vi "Automatic_IV_CV_with_XML_Global_Stop_V1.0.vi"() -> ()   [LabVIEW 2009]
uses:
  subVIs/CMSFPIX_LV80.llb/Keith 237 Operate/Standby.vi
  <vilib>/xml/Close Reference(Node).vi
  <vilib>/Utility/file.llb/Write To Spreadsheet File (string).vi
  <vilib>/Utility/file.llb/Write To Spreadsheet File (DBL).vi
  <vilib>/xml/NI_XML.lvlib
panel:
  out "voltage \ncompliance level":dbl=1e-05
  out "Wafer Number":string
  out "Contact Check Result":string="Skipped"
  out "Site Number":i32
  out "File Name":string
  in  "Tab Control 2":enum32{"IV Check", "CV Check"}(tab)
  out "Boolean":bool caption="Voltage Breakdown"
  out "Boolean 2":bool caption="Leakage Current Check Total"
  out "Boolean 3":bool caption="Leakage Current Check Active"
  out "Boolean 4":bool caption="Leakage Current Check Guardring"
  out "Boolean 5":bool caption="150V Bias Check"
  out "Contact Check":bool
  out "Status":string
  out "Bias Polarity":dbl=1.0 format="%.2f"
  out "1/C^2":cluster{"Y":dbl[], "Y":dbl[]}[](graph)
  out "semaphore":T1
  out "voltage \ncompliance cutoff":dbl=1e-05
  in  "Tab Control":enum32{"Site Selection"}(tab)
  in  "Site 1":bool=TRUE
  in  "Site 2":bool=TRUE
  in  "Site 3":bool=TRUE
  in  "Site 4":bool=TRUE
  in  "Site 5":bool=TRUE
  in  "Site 6":bool=TRUE
  in  "Site 7":bool=TRUE
  in  "Site 8":bool=TRUE
  in  "Site 9":bool=TRUE
  in  "Site 10":bool=TRUE
  in  "Site 11":bool=TRUE
  in  "Site 12":bool=TRUE
  in  "Site 13":bool=TRUE
  in  "Site 14":bool=TRUE
  in  "Site 15":bool=TRUE
  in  "Site 16":bool=TRUE
  in  "Site 17":bool=TRUE
  in  "Site 18":bool=TRUE
  in  "Site 19":bool=TRUE
  in  "Site 20":bool=TRUE
  in  "Site 21":bool=TRUE
  in  "Site 22":bool=TRUE
  in  "Running Conditional":bool
  out "error out 7":T2
  in  "IV or CV":i32
  in  "Emergency Stop":bool
  out "error out 6":T2
  in  "Stop Loop":bool=TRUE
  in  "Total Site # CV":i32=12
  out "Secondary Parameter":u16(ring) items=["None", "Cs", "Cp", "Ls", "Lp", "Rs", "Rp", "DF", "Q", "Z", "Y", "Phase", "ESR", "Gp", "Xs", "Bp"]
  out "Auto Compliance":dbl=9.9e-05
  out "Compliance":dbl=1e-09
  out "Compliance":bool
  out "Compliance Level":dbl format="%#_6e"
  out "Secondary Parameter Graph":cluster{"Y":dbl[], "Y":dbl[]}[](graph) caption="DF"
  in  "Absolute?":bool
  out "Voltage Range":string
  out "Primary Parameter":u16(ring)=2 items=["AUTO", "Cs", "Cp", "Ls", "Lp", "Rs", "Rp", "DF", "Q", "Z", "Y", "Phase", "ESR", "Gp", "Xs", "Bp"]
  out "Time Delay mS":dbl=20.0
  out "Number of Averages":dbl=1.0
  out "Voltage Level":dbl=1.0
  out "Frequency":dbl=1000.0
  in  "Bias Loop":bool
  out "K237_Bias":dbl
  in  "Archive":T3(tab)=enum."Primary"
  out "Diode Total Current Archive":cluster{"Y":dbl[], "Y":dbl[]}[](graph) caption="Total Current"
  out "Diode GRD Archive":cluster{"Y":dbl[], "Y":dbl[]}[](graph)
  out "Diode ACTIVE Archive":cluster{"Y":dbl[], "Y":dbl[]}[](graph)
  out "Single Chip Total Current Archive":cluster{"Y":dbl[], "Y":dbl[]}[](graph) caption="Total Current"
  out "Single Chip GRD Archive":cluster{"Y":dbl[], "Y":dbl[]}[](graph)
  out "Single Chip ACTIVE Archive":cluster{"Y":dbl[], "Y":dbl[]}[](graph)
  out "2x8 Total Current Archive":cluster{"Y":dbl[], "Y":dbl[]}[](graph) caption="Total Current"
  out "2x8 GRD Archive":cluster{"Y":dbl[], "Y":dbl[]}[](graph)
  out "2x8 ACTIVE Archive":cluster{"Y":dbl[], "Y":dbl[]}[](graph)
  out "Slim-Edge ACTIVE Archive":cluster{"Y":dbl[], "Y":dbl[]}[](graph)
  out "Slim-Edge GRD Archive":cluster{"Y":dbl[], "Y":dbl[]}[](graph)
  out "Slim-Edge Total Current Archive":cluster{"Y":dbl[], "Y":dbl[]}[](graph) caption="Total Current"
  out "Single Chip Capacitance":cluster{"Y":dbl[], "Y":dbl[]}[](graph)
  out "2x8 Chip Capacitance":cluster{"Y":dbl[], "Y":dbl[]}[](graph)
  out "Diodes Capacitance":cluster{"Y":dbl[], "Y":dbl[]}[](graph)
  in  "Halt CV":bool
  in  "Halt IV":bool
  out "Running?":bool
  in  "Total Site # IV":i32=22
  out "Site # CV":dbl
  out "Site # IV":dbl
  out "error out":errorcluster
  in  "CV-V-Limit":i32=10
  out "Capacitance":cluster{"Y":dbl[], "Y":dbl[]}[](graph) caption="Cp"
  in  "CV-V-Steps":i32=1
  out "QuadTech Status":string
  out "Total Current":cluster{"Y":dbl[], "Y":dbl[]}[](graph)
  out "6485 GRD (GPIB 10)":cluster{"Y":dbl[], "Y":dbl[]}[](graph)
  out "6485 ACTIVE (GPIB 14)":cluster{"Y":dbl[], "Y":dbl[]}[](graph)
  out "error out 5":errorcluster
  out "error out 4":errorcluster
  in  "IV-V-Steps":i32=1
  in  "IV-V-Limit":i32=10
  in  "error in (no error)":errorcluster
  # "Note: The Total Site # indexes\nstarting at 0 and goes to n-1,\nso if there are a total of 3 sites\nthen Total Site # should be set\nto 3"
  # "Note 2: This code is setup for a specific\nwafer map. If a map with a different\nnumber of subsites and/or different layout\nis used the naming will be incorrect"
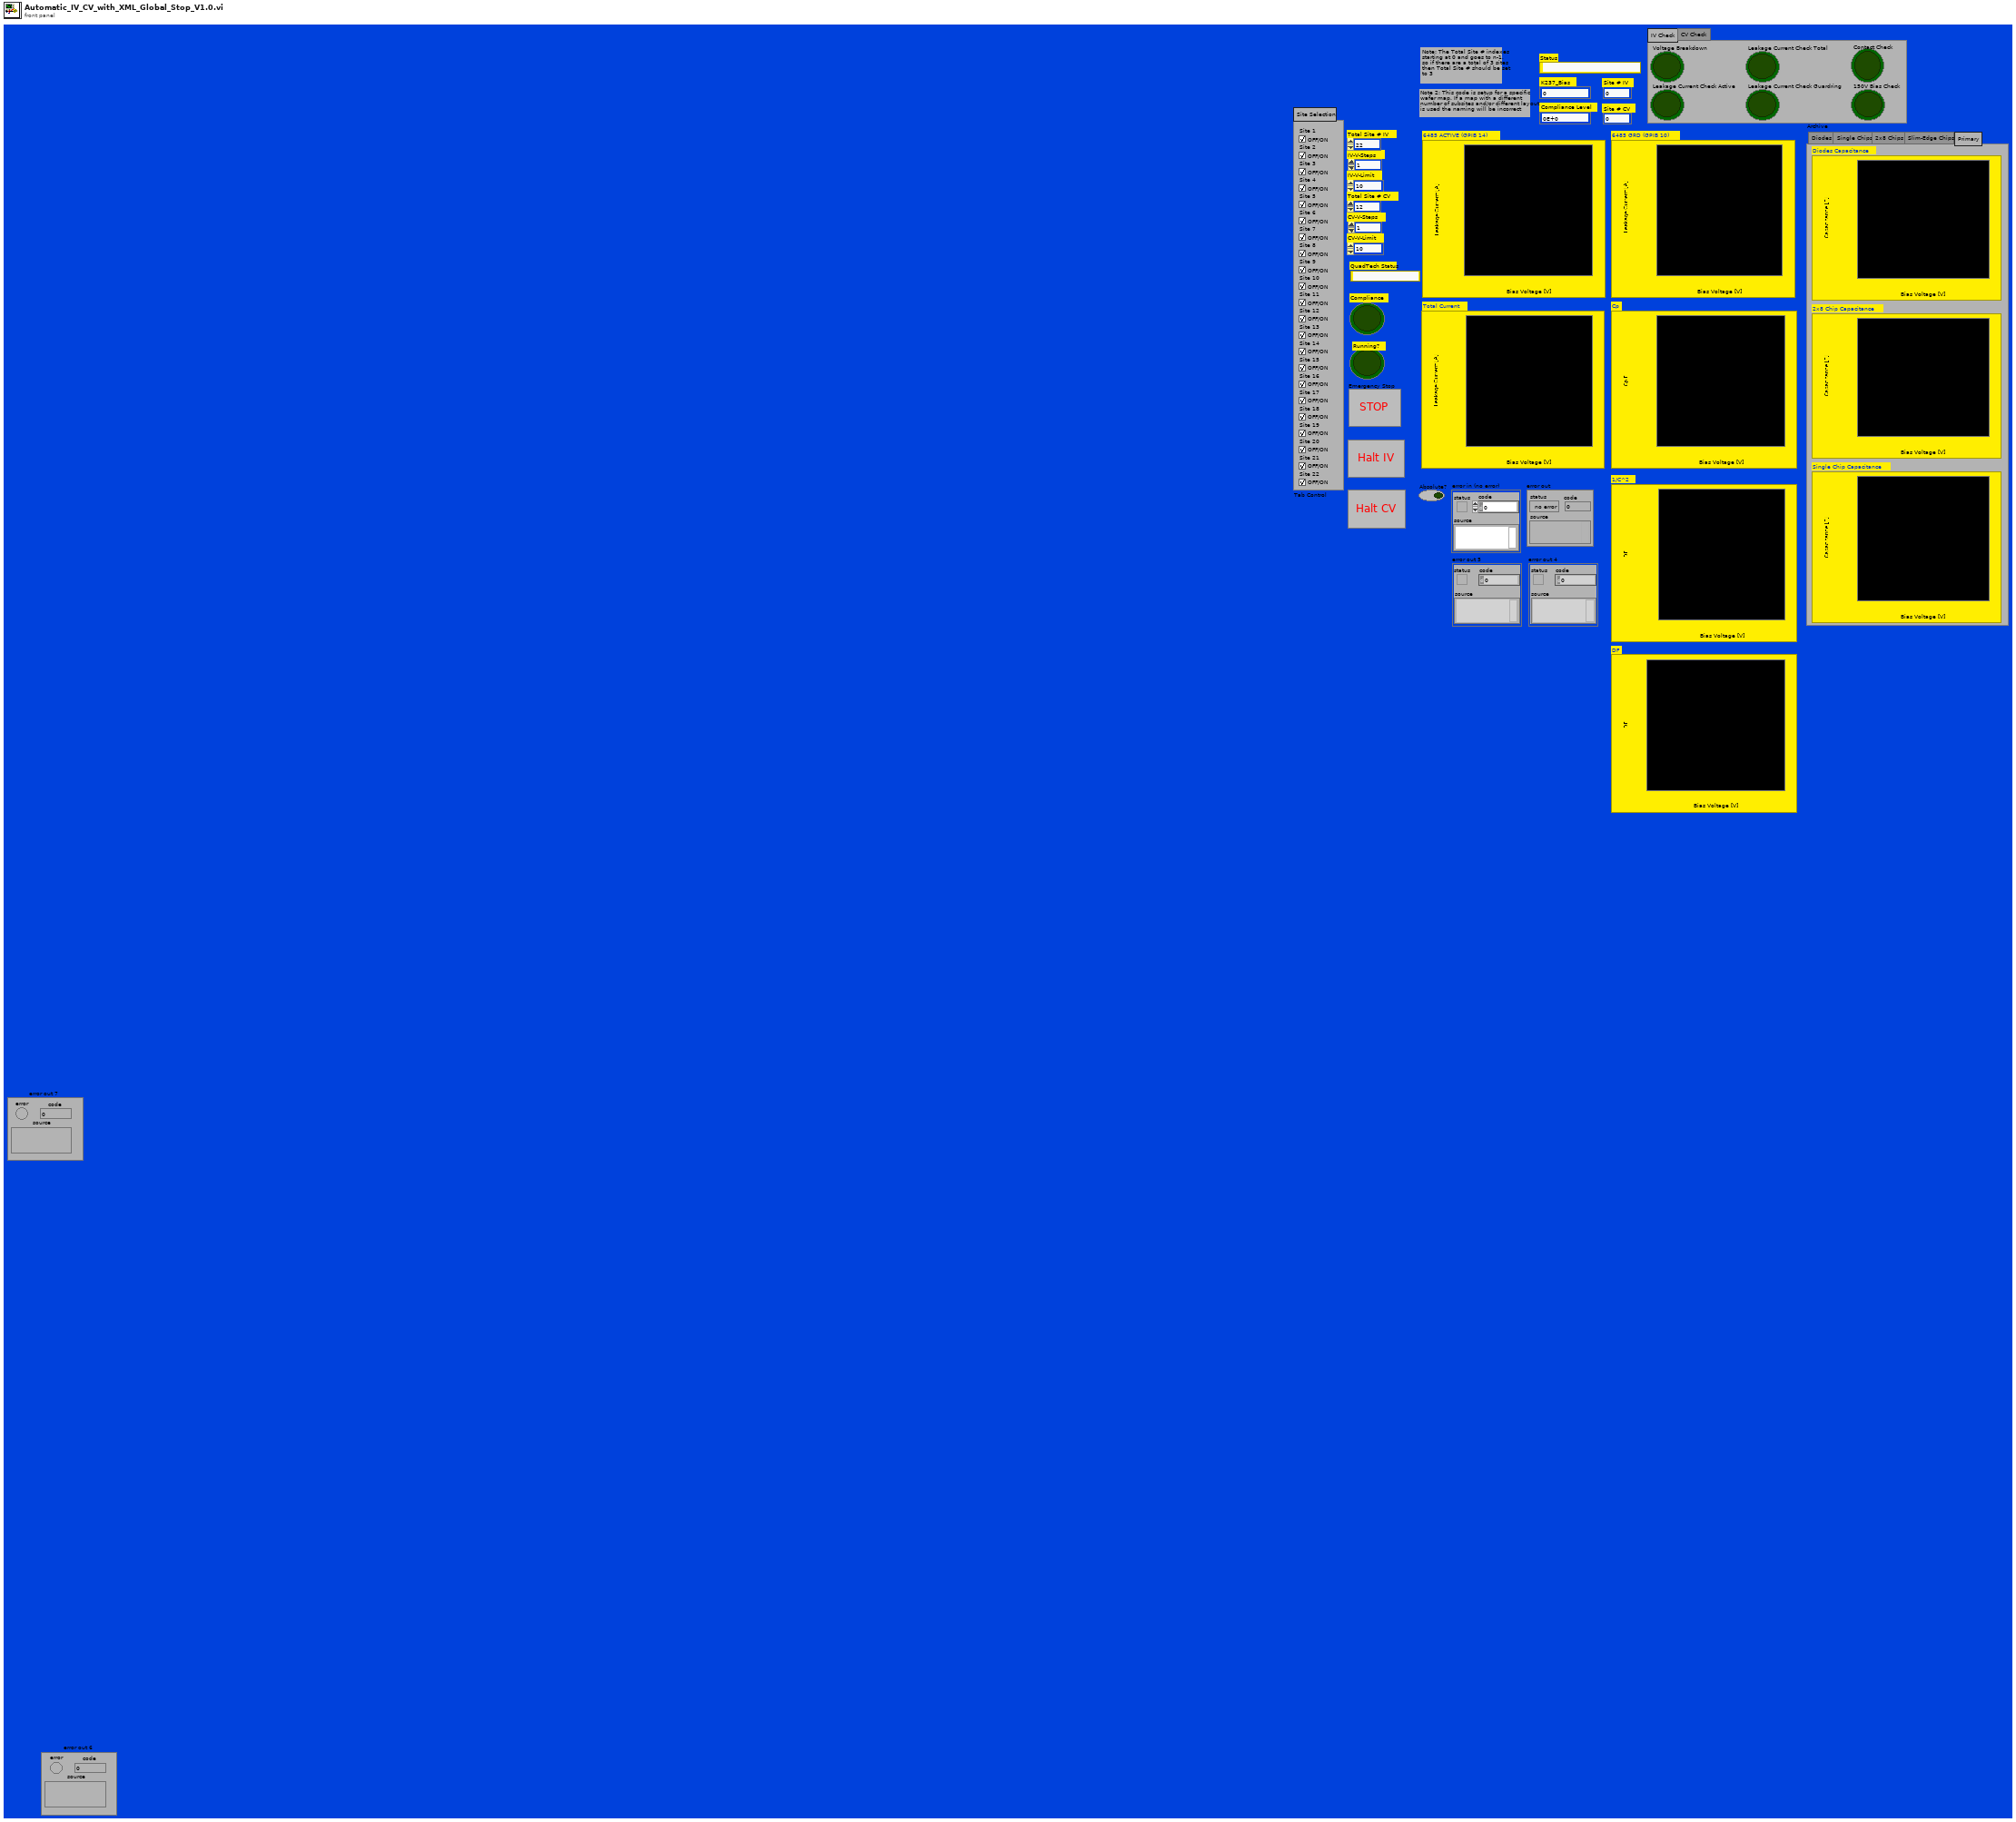
[diagram p1: front panel]
types:
  T1 = typedef "Semaphore RefNum" = refnum<k1>
  T2 = cluster{"error":bool, "code":i32, "source":string}
  T3 = enum32{"Diodes", "Single Chips", "2x8 Chips", "Slim-Edge Chips", "Primary"}
  T4 = cluster{"Name of Test":string, string, "Comment Description":string, "User":string}
  T5 = enum16{"open", "replace", "create", "open or create", "replace or create", "replace or create with confirmation"}
  T6 = cluster{cluster{"Y":dbl[], "Y":dbl[]}[], cluster{"Y":dbl[], "Y":dbl[]}[], cluster{"Y":dbl[], "Y":dbl[]}[], cluster{"Y":dbl[], "Y":dbl[]}[], cluster{"Y":dbl[], "Y":dbl[]}[], cluster{"Y":dbl[], "Y":dbl[]}[], cluster{"Y":dbl[], "Y":dbl[]}[], cluster{"Y":dbl[], "Y":dbl[]}[], cluster{"Y":dbl[], "Y":dbl[]}[], cluster{"Y":dbl[], "Y":dbl[]}[], cluster{"Y":dbl[], "Y":dbl[]}[], cluster{"Y":dbl[], "Y":dbl[]}[]}
  T7 = enum16{"Left Button", "Center Button", "Right Button", "Window Close"}
  T8 = cluster{"error":bool, "code":i8, "source":string}
  T9 = cluster{cluster{"Y":dbl[], "Y":dbl[]}[], cluster{"Y":dbl[], "Y":dbl[]}[], cluster{"Y":dbl[], "Y":dbl[]}[]}
  T10 = cluster{"Primary ":string, "Primary Value":string, "Primary Unit":string, "Secondary":string, "Secondary Value":string, "Secondary Unit":string}
  T11 = cluster{"XY Graph":cluster{"Y":dbl[], "Y":dbl[]}[], "XY Graph":cluster{"Y":dbl[], "Y":dbl[]}[], "XY Graph":cluster{"Y":dbl[], "Y":dbl[]}[]}
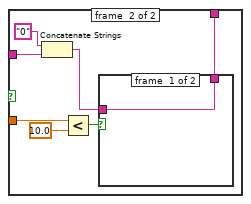
[diagram p4: hidden frame]
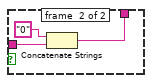
[diagram p5: hidden frame]
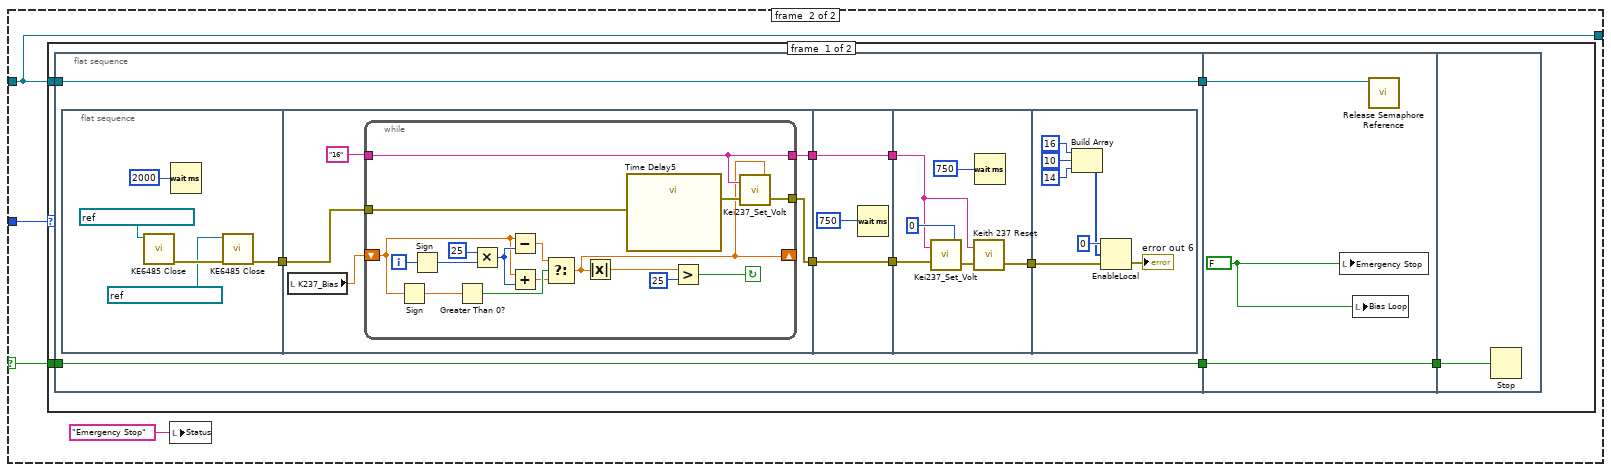
[diagram p7: hidden frame]
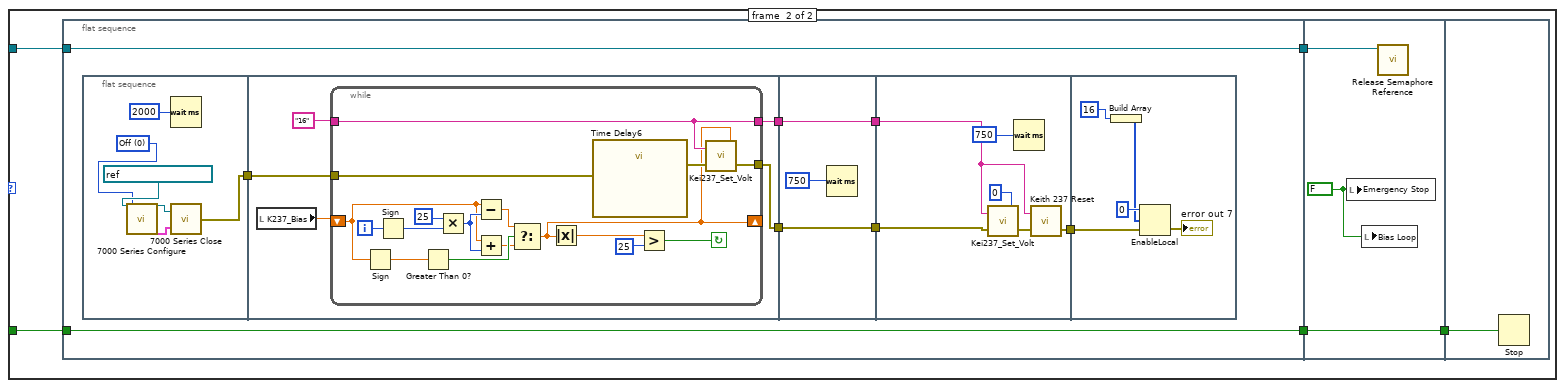
[diagram p8: hidden frame]
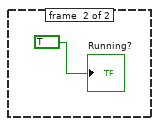
[diagram p9: hidden frame]
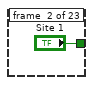
[diagram p10: hidden frame]
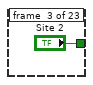
[diagram p11: hidden frame]
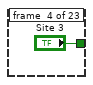
[diagram p12: hidden frame]
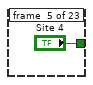
[diagram p13: hidden frame]
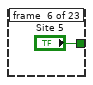
[diagram p14: hidden frame]
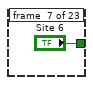
[diagram p15: hidden frame]
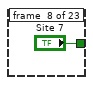
[diagram p16: hidden frame]
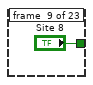
[diagram p17: hidden frame]
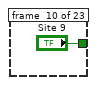
[diagram p18: hidden frame]
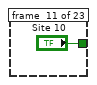
[diagram p19: hidden frame]
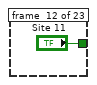
[diagram p20: hidden frame]
diagram:
  (unwired) path "" ("base path")
  # "Wafer Folder"
  # "Test Name Subfolder"
  # "XML Subfolder"
  # "Single Chip"
  # "2x8"
  # "Diode"
  # "Total"
  # "GRD"
  # "Active"
  # "Capacitance"
  # "Slim-Edge"
  # "2x8"
  # "Single Chip"
  # "Diodes"
  # "Change wiring to CV"
  # "DO CV MEASUREMENTS"
  # "Do CV measurements"
  # "Configure CV instuments"
  # "Do IV measurements"
  # "Configure IV instuments"
  # "DO IV MEASUREMENTS"
  n1 = invoke on="Diode ACTIVE Archive" class="XYGraph (strict)" method="Reinit To Default"() -> ()  [unwired: 3 in, 3 out]
  n2 = invoke on="Diode GRD Archive" class="XYGraph (strict)" method="Reinit To Default"() -> ()  [unwired: 3 in, 3 out]
  n3 = invoke on="Diode Total Current Archive" class="XYGraph (strict)" method="Reinit To Default"() -> ()  [unwired: 3 in, 3 out]
  n4 = invoke on="Diodes Capacitance" class="XYGraph (strict)" method="Reinit To Default"() -> ()  [unwired: 3 in, 3 out]
  n5 = invoke on="2x8 Chip Capacitance" class="XYGraph (strict)" method="Reinit To Default"() -> ()  [unwired: 3 in, 3 out]
  n6 = invoke on="Single Chip Capacitance" class="XYGraph (strict)" method="Reinit To Default"() -> ()  [unwired: 3 in, 3 out]
  n7 = invoke on="Single Chip ACTIVE Archive" class="XYGraph (strict)" method="Reinit To Default"() -> ()  [unwired: 3 in, 3 out]
  n8 = invoke on="Single Chip GRD Archive" class="XYGraph (strict)" method="Reinit To Default"() -> ()  [unwired: 3 in, 3 out]
  n9 = invoke on="Single Chip Total Current Archive" class="XYGraph (strict)" method="Reinit To Default"() -> ()  [unwired: 3 in, 3 out]
  n10 = invoke on="2x8 ACTIVE Archive" class="XYGraph (strict)" method="Reinit To Default"() -> ()  [unwired: 3 in, 3 out]
  n11 = invoke on="2x8 GRD Archive" class="XYGraph (strict)" method="Reinit To Default"() -> ()  [unwired: 3 in, 3 out]
  n12 = invoke on="2x8 Total Current Archive" class="XYGraph (strict)" method="Reinit To Default"() -> ()  [unwired: 3 in, 3 out]
  n13 = local write "K237_Bias"(0.0 ("K237_Bias")) -> ()
  n14 = invoke on="Slim-Edge ACTIVE Archive" class="XYGraph (strict)" method="Reinit To Default"() -> ()  [unwired: 3 in, 3 out]
  n15 = invoke on="Slim-Edge GRD Archive" class="XYGraph (strict)" method="Reinit To Default"() -> ()  [unwired: 3 in, 3 out]
  n16 = invoke on="Slim-Edge Total Current Archive" class="XYGraph (strict)" method="Reinit To Default"() -> ()  [unwired: 3 in, 3 out]
  n17 = call "Wafer ID"("error in (no error)"="error in (no error)") -> ("User"=w20:string, "Comment Description"=w21:string, "Name of Test"=w3:string, "Wafer ID #"=w14:dbl, "OK"=w62:bool, "error out"=w65:errorcluster)  [unwired: 13 in]
  n18 = Number To Decimal String(number=w14) -> (decimal integer string=w15:string)  [unwired: 1 in]
  n19 = Less?(x=w14, y=100.0) -> (x < y?=w17:bool)
  n20 = case shown="True" w17 {
    tunnel: w15 -> [w67 w74]
    tunnel: w14 -> [_ w71]
    tunnel: [w67 w68] -> w13
    frame #0 {
    }
    frame #1 {
      n21 = Concatenate Strings("0" ("string"), w74) -> (w69:string)
      n22 = Less?(x=w71, y=10.0) -> (x < y?=w72:bool)
      n23 = case shown="True" w72 {
        tunnel: w69 -> [w75 w78]
        tunnel: [w75 w76] -> w68
        frame #0 {
        }
        frame #1 {
          n24 = Concatenate Strings("0" ("string"), w78) -> (w76:string)
        }
      }
    }
  }
  "Wafer Number" <- w13
  n25 = Not(x=w62) -> (.not. x?=w61:bool)
  n26 = call <vilib>:"Obtain Semaphore Reference.vi"("size (1)"=1) -> ("semaphore"=w34:T1)  [unwired: 4 in, 2 out]
  "semaphore" <- w34
  n27 = Stop(stop? (T)=w61) -> ()
  n28 = Concatenate Strings("Wafer_" ("string"), w13) -> (w25:string)
  n29 = Build Path(base path=path "C:/Documents and Settings/PROBER/Desktop/Andrew_Test/VI Test Output", name or relative path=w25) -> (appended path=w24:path)
  n30 = Bundle("Name of Test"=w3, w13, "Comment Description"=w21, "User"=w20) -> (w12:T4)  [unwired: 1 in]
  n31 = flat-sequence {
    tunnel: w65 -> [w99]
    tunnel: [w97] -> w64
    tunnel: [w85] -> w58
    tunnel: [w87] -> w57
    tunnel: [w86] -> w56
    tunnel: [w90] -> w35
    tunnel: w34 -> [w90]
    tunnel: [w80] -> w18
    tunnel: w64 -> [w138]
    tunnel: w1 -> [w133]
    tunnel: w58 -> [w131]
    tunnel: w57 -> [w130]
    tunnel: w56 -> [w129]
    tunnel: [w128] -> w45
    tunnel: w35 -> [w121]
    tunnel: [w120] -> w28
    tunnel: w12 -> [w119]
    tunnel: w18 -> [w118]
    tunnel: w1 -> [w113]
    tunnel: w7 -> [w111]
    tunnel: w45 -> [w1215]
    tunnel: [w1215] -> w44
    tunnel: [w1213] -> w29
    tunnel: w28 -> [w1213]
    tunnel: [w1219] -> w46
    tunnel: w44 -> [w1220]
    tunnel: [w1217] -> w30
    tunnel: w29 -> [w1217]
    tunnel: w46 -> [w1229]
    tunnel: [w1229] -> w63
    tunnel: [w1225] -> w31
    tunnel: w30 -> [_]
    tunnel: w63 -> [w1238]
    tunnel: [w1237] -> w55
    tunnel: [w1236] -> w53
    tunnel: [w1235] -> w51
    tunnel: [w1233] -> w49
    tunnel: [w1232] -> w32
    tunnel: w31 -> [w1232]
    tunnel: w55 -> [w1272]
    tunnel: [w1272] -> w54
    tunnel: w53 -> [w1271]
    tunnel: [w1271] -> w52
    tunnel: w51 -> [w1270]
    tunnel: [w1270] -> w50
    tunnel: w49 -> [w1269]
    tunnel: ["Total Site # CV"] -> w37
    tunnel: [w1267] -> w33
    tunnel: w32 -> [w1267]
    tunnel: w54 -> [w1320]
    tunnel: w52 -> [w1319]
    tunnel: w50 -> [w1318]
    tunnel: w1 -> [w1310]
    tunnel: [FALSE ("Compliance")] -> w43
    tunnel: [TRUE ("Bias Loop")] -> w41
    tunnel: [w1308] -> w39
    tunnel: w37 -> [w1307]
    tunnel: w33 -> [w1306]
    tunnel: w12 -> [w1304]
    tunnel: w7 -> [w1303]
    tunnel: w43 -> [w1874]
    tunnel: [w1874] -> w42
    tunnel: w41 -> [w1877]
    tunnel: [w1877] -> w40
    tunnel: w39 -> [w1876]
    tunnel: [w1876] -> w38
    tunnel: [w1885] -> w47
    tunnel: [w1886] -> w48
    tunnel: w42 -> [w1886]
    tunnel: w40 -> [w1885]
    tunnel: w38 -> [w1880]
    frame #0 {
      w80 = 0 ("Numeric")
      w91 = FALSE
      w100 = u16 5 items=["auto / auto", "1 nA / 1.1 V", "10 nA / 11 V", "100 nA / 110 V", "0.001 mA / 1100 V", "0.01 mA / 1100 V", "0.1 mA / 1100 V", "1 mA / 1100 V", "10 mA / 1100 V", "100 mA / 1100 V"] ("source range\nI source / V source (auto:0)")
      w103 = u16 0 items=["voltage/current", "current/voltage"] ("source/measure (V/I:0)")
      w104 = u16 5 items=["auto / auto", "1 nA / 1.1 V", "10 nA / 11 V", "100 nA / 110 V", "0.001 mA / 1100 V", "0.01 mA / 1100 V", "0.1 mA / 1100 V", "1 mA / 1100 V", "10 mA / 1100 V", "100 mA / 1100 V"] ("compliance/\nmeasurement range (auto:0)")
      w102 = 1e-05 ("voltage \ncompliance level")
      w107 = u16 0 items=["DC", "sweep"] ("function (DC:0)")
      w97 = "16"  # GPIB
      # "Change Bias Polarity\n+1 Chuck Bias\n-1  Pad bias"
      # "Keithley 237 as sourcemeter\nKeithley 6485 as picoammeters"
      n32 = call "Keith 237 Reset.vi"("GPIB address"=w97, "error in"=w99) -> ("error out"=w98:T2)
      n33 = call "Keith 237 Basic Config.vi"("GPIB address"=w97, "source/measure (V/I:0)"=w103, "function (DC:0)"=w107, "source range\nI source / V source (auto:0)"=w100, "source level"=0.0, "error in"=w98, "1100 V range (disabled:F)"=TRUE, "current \ncompliance level"=w102, "compliance/\nmeasurement range (auto:0)"=w104) -> ("error out"=w109:T2)  [unwired: 7 in, 3 out]
      n34 = local write "IV or CV"(w80) -> ()
      n35 = call "Keith 237 Operate/Standby.vi"("source"=FALSE, "error in"=w109, "GPIB address"=w97) -> ("error out"=w108:T2)
      n36 = Multiply(x=w102, y=0.98 ("voltage \ncompliance level")) -> (x*y=→"voltage \ncompliance cutoff":dbl)
      n37 = call "Keith 237 Send Trigger.vi"("GPIB address"=w97, "error in"=w108) -> ("error out"=w95:T2)
      n38 = call "KE6485 Initialize.vi"("error in (no error)"=w95, "resource name"=refnum<k15> "GPIB0::10::INSTR" ("instrument handle")) -> ("error out"=w89:errorcluster, "instrument handle out"=w92:refnum<k15>)  [unwired: 8 in]
      n39 = property class="KE6485"(reference=w92, error in=w89, "System Settings:Zero Check Enabled"=w91) -> (reference out=w85:refnum<k15>, error out=w84:errorcluster)
      n40 = call "KE6485 Initialize.vi"("error in (no error)"=w84, "resource name"=refnum<k15> "GPIB0::14::INSTR" ("instrument handle")) -> ("error out"=w88:errorcluster, "instrument handle out"=w93:refnum<k15>)  [unwired: 8 in]
      n41 = property class="KE6485"(reference=w93, error in=w88, "System Settings:Zero Check Enabled"=w91) -> (reference out=w87:refnum<k15>, error out=w86:errorcluster)
      "Bias Polarity" <- 1.0
      "Status" <- "Setting IV Scan Parameters" ("Status")
      "voltage \ncompliance level" <- w102
    }
    frame #1 {
      w122 = cluster{"Y":dbl[], "Y":dbl[]}[] []
      # "10"
      # "14"
      n42 = Build Path(base path=w113, name or relative path="Contact_Check.csv") -> (appended path=w117:path)
      n43 = Open/Create/Replace File(file path (use dialog)=w117, operation (0:open)=T5."replace or create", access (0:read/write)=enum16{"read/write", "read-only", "write-only"}."read/write") -> (refnum out=w116:refnum<file>)  [unwired: 1 in, 4 out]
      n44 = Refnum to Path(1:w116) -> (0:w112:path)
      n45 = for {
        N: "Total Site # IV" -> [_]
        tunnel: w138 -> [w232]
        tunnel: "IV-V-Limit" -> [w234]
        tunnel: "IV-V-Steps" -> [w235]
        tunnel: [w231] -> w136
        shift-right: [w230] -> w124
        shift-left: w129 -> [w233]
        shift-right: [w225] -> _
        shift-left: w122 -> [w196]
        shift-right: [w224] -> _
        shift-left: w122 -> [w195]
        shift-right: [w223] -> _
        shift-left: w122 -> [w194]
        shift-right: [w222] -> _
        shift-left: w122 -> [w193]
        shift-right: [w221] -> _
        shift-left: w122 -> [w188]
        shift-right: [w220] -> _
        shift-left: w122 -> [w192]
        shift-right: [w219] -> _
        shift-left: w122 -> [w191]
        shift-right: [w199] -> _
        shift-left: w122 -> [w190]
        shift-right: [w218] -> _
        shift-left: w122 -> [w189]
        tunnel: w133 -> [w201]
        tunnel: "Absolute?" -> [w200]
        tunnel: w131 -> [w198]
        tunnel: w130 -> [w197]
        shift-right: [w183] -> _
        shift-left: w122 -> [w186]
        shift-right: [w182] -> _
        shift-left: w122 -> [w185]
        shift-right: [w181] -> _
        shift-left: w122 -> [w184]
        tunnel: w121 -> [w180]
        tunnel: [w179] -> w120
        tunnel: w119 -> [w164]
        tunnel: w118 -> [w166]
        tunnel: w112 -> [w142]
        tunnel: w111 -> [w140]
        i -> [w165]
        (unwired) TRUE
        # "User Input Array\nElement 0: Comment Description (XML_Header)\nElement 1: Serial Number\nElement 2: Kind of Part\nElement 3: User\nElement 4: Extension Table Name\nElement 5: Comment Description (XML_Data_Set)\nElement 6: Name (XML_Header)\nElement 7: Run Name (XML_Header)"
        # "XML Data Tags for IV scan"
        n46 = Increment(x=w165) -> (x+1=→"Site # IV":i32)
        n47 = Bundle(w196, w195, w194, w193, w192, w191, w190, w189, w188, w186, w185, w184) -> (w187:T6)  [unwired: 1 in]
        n48 = flat-sequence {
          tunnel: [w246] -> w150
          tunnel: w233 -> [w246]
          tunnel: [w245] -> w152
          tunnel: w232 -> [w245]
          tunnel: w165 -> [w237]
          tunnel: [w244] -> w154
          tunnel: w198 -> [w244]
          tunnel: [w243] -> w156
          tunnel: w197 -> [w243]
          tunnel: w180 -> [w242]
          tunnel: [w242] -> w158
          tunnel: [w236] -> w148
          tunnel: [w238] -> w147
          tunnel: [w240] -> w145
          tunnel: [w237] -> w141
          tunnel: w158 -> [w288]
          tunnel: [w287] -> w157
          tunnel: w156 -> [w286]
          tunnel: [w285] -> w155
          tunnel: w154 -> [w284]
          tunnel: [w283] -> w153
          tunnel: w152 -> [w281]
          tunnel: [w280] -> w151
          tunnel: w150 -> [w282]
          tunnel: [w279] -> w149
          tunnel: w148 -> [w271]
          tunnel: w147 -> [w275]
          tunnel: [w275] -> w146
          tunnel: w145 -> [w276]
          tunnel: [w276] -> w144
          tunnel: [w278] -> w143
          tunnel: w141 -> [w272]
          tunnel: w235 -> [w540]
          tunnel: w234 -> [w539]
          tunnel: [w536] -> w207
          tunnel: [w535] -> w206
          tunnel: [w528] -> w205
          tunnel: [w534] -> w204
          tunnel: [w533] -> w203
          tunnel: w217 -> [w532]
          tunnel: w168 -> [w530]
          tunnel: w208 -> [w529]
          tunnel: [w524] -> w202
          tunnel: w200 -> [w527]
          tunnel: [w522] -> w179
          tunnel: w157 -> [w523]
          tunnel: w155 -> [w525]
          tunnel: w153 -> [w526]
          tunnel: w151 -> [w537]
          tunnel: w149 -> [w538]
          tunnel: w146 -> [w517]
          tunnel: w144 -> [w515]
          tunnel: w159 -> [w521]
          tunnel: w139 -> [w520]
          tunnel: w160 -> [w519]
          tunnel: w143 -> [w518]
          tunnel: w139 -> [w513]
          tunnel: w207 -> [w914]
          tunnel: [w913] -> w178
          tunnel: w206 -> [w910]
          tunnel: [w912] -> w176
          tunnel: w205 -> [w917]
          tunnel: [w917] -> w174
          tunnel: w204 -> [w916]
          tunnel: [w916] -> w172
          tunnel: w203 -> [w915]
          tunnel: [w915] -> w170
          tunnel: w202 -> [w911]
          tunnel: w178 -> [w946]
          tunnel: [w946] -> w177
          tunnel: w176 -> [w945]
          tunnel: [w945] -> w175
          tunnel: w174 -> [w944]
          tunnel: [w944] -> w173
          tunnel: w172 -> [w943]
          tunnel: [w943] -> w171
          tunnel: w170 -> [w942]
          tunnel: [w942] -> w169
          tunnel: [w967] -> w230
          tunnel: [w969] -> w231
          tunnel: w177 -> [w969]
          tunnel: w175 -> [w1006]
          tunnel: w165 -> [w1001]
          tunnel: w173 -> [w1000]
          tunnel: w171 -> [w999]
          tunnel: w169 -> [w998]
          tunnel: [w997] -> w225
          tunnel: [w996] -> w224
          tunnel: [w995] -> w223
          tunnel: [w994] -> w222
          tunnel: [w993] -> w221
          tunnel: [w992] -> w220
          tunnel: [w991] -> w219
          tunnel: [w990] -> w199
          tunnel: [w989] -> w218
          tunnel: w187 -> [w987]
          tunnel: [w973] -> w183
          tunnel: [w972] -> w182
          tunnel: [w971] -> w181
          tunnel: w142 -> [w951]
          frame #0 {
            n49 = Increment(x=w237) -> (x+1=w241:i32)
            n50 = case shown="1" w241 {
              tunnel: [TRUE "Site 1" "Site 2" "Site 3" "Site 4" "Site 5" "Site 6" "Site 7" "Site 8" "Site 9" "Site 10" "Site 11" "Site 12" "Site 13" "Site 14" "Site 15" "Site 16" "Site 17" "Site 18" "Site 19" "Site 20" "Site 21" "Site 22"] -> w238
              frame #0 {
              }
              frame #1 {
              }
              frame #2 {
              }
              frame #3 {
              }
              frame #4 {
              }
              frame #5 {
              }
              frame #6 {
              }
              frame #7 {
              }
              frame #8 {
              }
              frame #9 {
              }
              frame #10 {
              }
              frame #11 {
              }
              frame #12 {
              }
              frame #13 {
              }
              frame #14 {
              }
              frame #15 {
              }
              frame #16 {
              }
              frame #17 {
              }
              frame #18 {
              }
              frame #19 {
              }
              frame #20 {
              }
              frame #21 {
              }
              frame #22 {
              }
            }
            n51 = Wait (ms)(milliseconds to wait=u32 250) -> ()  [unwired: 1 out]
            n52 = Increment(x=w237) -> (x+1=w236:i32)
            n53 = call "Skip Current Subsite"("Enable"=w238) -> ("Skip Subsite"=w240:bool)  [unwired: 17 in, 1 out]
          }
          frame #1 {
            w270 = FALSE ("Visible")
            n54 = local write "Boolean"(w270) -> ()
            n55 = local write "Boolean 2"(w270) -> ()
            n56 = local write "Boolean 3"(w270) -> ()
            n57 = local write "Boolean 4"(w270) -> ()
            n58 = local write "Boolean 5"(w270) -> ()
            n59 = local write "Contact Check"(w270) -> ()
            n60 = Not(x=w275) -> (.not. x?=w274:bool)
            n61 = property on="Tab Control 2" class="TabCtl (strict)"("Visible"=TRUE) -> ()  [unwired: 2 in, 2 out]
            n62 = Compound Arithmetic op=OR(w274, w276) -> (w277:bool)
            n63 = case shown="False" w277 {
              tunnel: w288 -> [w301 w508]
              tunnel: [w300 w508] -> w287
              tunnel: w286 -> [w299 w509]
              tunnel: [w298 w509] -> w285
              tunnel: w284 -> [w297 w510]
              tunnel: [w296 w510] -> w283
              tunnel: w271 -> [w295 w506]
              tunnel: w282 -> [w294 w511]
              tunnel: w281 -> [w293 w512]
              tunnel: [w292 w512] -> w280
              tunnel: [w291 w511] -> w279
              tunnel: [w290 TRUE] -> w278
              tunnel: w272 -> [w289 _]
              frame #0 {
                n64 = flat-sequence {
                  tunnel: w301 -> [w317]
                  tunnel: w299 -> [w316]
                  tunnel: w297 -> [w315]
                  tunnel: w295 -> [w312]
                  tunnel: [w317] -> w306
                  tunnel: [w316] -> w305
                  tunnel: [w315] -> w304
                  tunnel: [w311] -> w303
                  tunnel: w293 -> [w311]
                  tunnel: [w310] -> w302
                  tunnel: w294 -> [w310]
                  tunnel: w289 -> [w307]
                  tunnel: [w378] -> w296
                  tunnel: [w377] -> w298
                  tunnel: [w375] -> w300
                  tunnel: w306 -> [w376]
                  tunnel: w305 -> [w384]
                  tunnel: w304 -> [w383]
                  tunnel: w303 -> [w382]
                  tunnel: w302 -> [w381]
                  tunnel: [w380] -> w292
                  tunnel: [w379] -> w291
                  tunnel: [w321] -> w290
                  frame #0 {
                    # "Go to N subsite"
                    n65 = Number To Decimal String(number=w307) -> (decimal integer string=w314:string)  [unwired: 1 in]
                    n66 = local write "Contact Check Result"("Not Skipped" ("Contact Check Result")) -> ()
                    n67 = Wait (ms)(milliseconds to wait=u32 1500) -> ()  [unwired: 1 out]
                    n68 = call "-mov-prob-abs-subs.vi"("Subsite #"=w314) -> ()  [unwired: 5 in]
                    n69 = local write "Status"("Moving to Subsite" ("Status")) -> ()
                    "Site Number" <- w312
                  }
                  frame #1 {
                    # "Contact Check"
                    n70 = local read "Bias Polarity"() -> (w319:dbl)
                    n71 = Wait (ms)(milliseconds to wait=u32 500) -> ()  [unwired: 1 out]
                    n72 = local write "Status"("IV Contact Check" ("Status")) -> ()
                    n73 = Multiply(x=w319, y=3.0) -> (x*y=w318:dbl)
                    n74 = flat-sequence {
                      tunnel: w384 -> [w391]
                      tunnel: w383 -> [w392]
                      tunnel: w381 -> [w393]
                      tunnel: [w393] -> w374
                      tunnel: [w392] -> w373
                      tunnel: [w391] -> w372
                      tunnel: [w390] -> w371
                      tunnel: w376 -> [w389]
                      tunnel: w382 -> [w388]
                      tunnel: [w388] -> w370
                      tunnel: [w387] -> w369
                      tunnel: w318 -> [w387]
                      tunnel: w374 -> [w399]
                      tunnel: [w398] -> w368
                      tunnel: w373 -> [w402]
                      tunnel: [w402] -> w367
                      tunnel: w372 -> [w401]
                      tunnel: [w401] -> w366
                      tunnel: w371 -> [w400]
                      tunnel: [w400] -> w365
                      tunnel: w370 -> [w396]
                      tunnel: [w396] -> w364
                      tunnel: w369 -> [w395]
                      tunnel: [w394] -> w363
                      tunnel: [w409] -> w362
                      tunnel: [w407] -> w361
                      tunnel: [w406] -> w360
                      tunnel: w368 -> [w408]
                      tunnel: w367 -> [w407]
                      tunnel: w366 -> [w406]
                      tunnel: [w405] -> w359
                      tunnel: w365 -> [w405]
                      tunnel: [w404] -> w358
                      tunnel: w364 -> [w404]
                      tunnel: w363 -> [w403]
                      tunnel: w362 -> [w415]
                      tunnel: w361 -> [w414]
                      tunnel: w360 -> [w413]
                      tunnel: [w415] -> w357
                      tunnel: [w414] -> w356
                      tunnel: [w413] -> w355
                      tunnel: w359 -> [w412]
                      tunnel: [w411] -> w354
                      tunnel: [w410] -> w353
                      tunnel: w358 -> [w410]
                      tunnel: w357 -> [w418]
                      tunnel: w356 -> [w421]
                      tunnel: w355 -> [w420]
                      tunnel: [w417] -> w352
                      tunnel: [w421] -> w351
                      tunnel: [w420] -> w350
                      tunnel: [w419] -> w349
                      tunnel: w354 -> [w419]
                      tunnel: [w416] -> w348
                      tunnel: w353 -> [w416]
                      tunnel: w352 -> [w427]
                      tunnel: w351 -> [w426]
                      tunnel: w350 -> [w425]
                      tunnel: [w427] -> w347
                      tunnel: [w426] -> w346
                      tunnel: [w425] -> w345
                      tunnel: w349 -> [w424]
                      tunnel: [w423] -> w344
                      tunnel: [w422] -> w343
                      tunnel: w348 -> [w422]
                      tunnel: w347 -> [w437]
                      tunnel: w346 -> [w432]
                      tunnel: w345 -> [w431]
                      tunnel: [w434] -> w342
                      tunnel: [w433] -> w341
                      tunnel: w344 -> [w433]
                      tunnel: w343 -> [w430]
                      tunnel: [w432] -> w340
                      tunnel: [w431] -> w339
                      tunnel: [w430] -> w338
                      tunnel: [w429] -> w337
                      tunnel: [w428] -> w336
                      tunnel: w342 -> [w444]
                      tunnel: [w447] -> w335
                      tunnel: w341 -> [w450]
                      tunnel: [w450] -> w334
                      tunnel: w340 -> [w449]
                      tunnel: [w449] -> w333
                      tunnel: w339 -> [w448]
                      tunnel: [w448] -> w332
                      tunnel: w338 -> [w443]
                      tunnel: [w443] -> w331
                      tunnel: w337 -> [w441]
                      tunnel: [w440] -> w330
                      tunnel: w336 -> [w439]
                      tunnel: [w438] -> w329
                      tunnel: w335 -> [w458]
                      tunnel: w334 -> [w457]
                      tunnel: w333 -> [w455]
                      tunnel: w332 -> [w454]
                      tunnel: w331 -> [w453]
                      tunnel: [w458] -> w328
                      tunnel: [w456] -> w327
                      tunnel: [w455] -> w326
                      tunnel: [w454] -> w325
                      tunnel: [w453] -> w324
                      tunnel: w330 -> [w452]
                      tunnel: [w452] -> w323
                      tunnel: w329 -> [w451]
                      tunnel: [w451] -> w322
                      tunnel: [w467] -> w380
                      tunnel: [w468] -> w377
                      tunnel: [w469] -> w378
                      tunnel: [w470] -> w375
                      tunnel: [w471] -> w379
                      tunnel: w328 -> [w471]
                      tunnel: w327 -> [w470]
                      tunnel: w326 -> [w469]
                      tunnel: w325 -> [w468]
                      tunnel: w324 -> [w467]
                      tunnel: w323 -> [w463]
                      tunnel: w322 -> [w462]
                      tunnel: [w461] -> w321
                      frame #0 {
                        n75 = call <vilib>:"Acquire Semaphore.vi"("semaphore"=w389) -> ("semaphore out"=w390:T1)  [unwired: 4 in, 2 out]
                      }
                      frame #1 {
                        n76 = call "Keith 237 Operate/Standby.vi"("source"=TRUE, "error in"=w399, "GPIB address"=w396) -> ("error out"=w398:T2)
                        n77 = Negate(x=w395) -> (-x=w394:dbl)
                      }
                      frame #2 {
                        n78 = call "Kei237_Set_Volt.vi"("Voltage"=w403, "error in"=w408, "GPIB"=w404) -> ("error out"=w409:errorcluster)
                        n79 = local write "K237_Bias"(w403) -> ()
                      }
                      frame #3 {
                        n80 = call <vilib>:"Release Semaphore.vi"("semaphore"=w412) -> ("semaphore out"=w411:T1)  [unwired: 5 in, 1 out]
                      }
                      frame #4 {
                        n81 = call "Time Delay7"("error in (no error)"=w418) -> ("error out"=w417:errorcluster)  [unwired: 10 in]
                      }
                      frame #5 {
                        n82 = call <vilib>:"Acquire Semaphore.vi"("semaphore"=w424) -> ("semaphore out"=w423:T1)  [unwired: 4 in, 2 out]
                      }
                      frame #6 {
                        # "14"
                        # "10"
                        n83 = call "K237-read-current-2.vi"("error in"=w437, "GPIB"=w430) -> ("error out"=w436:T2)  [unwired: 1 out]
                        n84 = call "KE6485 Read.vi"("error in (no error)"=w436, "instrument handle"=w432) -> ("error out"=w435:errorcluster, "reading"=w429:dbl)  [unwired: 7 in, 1 out]
                        n85 = call "KE6485 Read.vi"("error in (no error)"=w435, "instrument handle"=w431) -> ("error out"=w434:errorcluster, "reading"=w428:dbl)  [unwired: 7 in, 1 out]
                      }
                      frame #7 {
                        n86 = call "Kei237_Set_Volt.vi"("Voltage"=0.0, "error in"=w444, "GPIB"=w443) -> ("error out"=w445:errorcluster)
                        n87 = Absolute Value(x=w439) -> (abs(x)=w438:dbl)
                        n88 = Absolute Value(x=w441) -> (abs(x)=w440:dbl)
                        n89 = call "Keith 237 Operate/Standby.vi"("source"=FALSE, "error in"=w445, "GPIB address"=w443) -> ("error out"=w447:T2)
                      }
                      frame #8 {
                        n90 = call <vilib>:"Release Semaphore.vi"("semaphore"=w457) -> ("semaphore out"=w456:T1)  [unwired: 5 in, 1 out]
                      }
                      frame #9 {
                        w464 = 1e-06
                        n91 = Greater?(x=w463, y=w464) -> (0:w466:bool)
                        n92 = Greater?(x=w462, y=w464) -> (0:w465:bool)
                        n93 = And(x=w466, y=w465) -> (x .and. y?=w460:bool)
                        "Contact Check" <- w460
                        n94 = local read "Site Number"() -> (w459:i32)
                        n95 = case shown="False" w460 {
                          tunnel: [w494 FALSE] -> w461
                          frame #0 {
                            (unwired) "Continue" ("Right Button Text (\"Cancel\")")
                            n96 = call <vilib>:"Three Button Dialog.vi"("Window Title (\"\")"="Contact Check Failed" ("Window Title (\"\")"), "Center Button Text (\"No\")"="Global Stop" ("Center Button Text (\"No\")"), "Left Button Text (\"Yes\")"="Skip Subsite" ("Left Button Text (\"Yes\")"), "message"="Warning: If the light needs to be turned on make sure the K237 is in Standby") -> ("Which Button?"=w495:T7)  [unwired: 7 in]
                            n97 = case shown="\"Right Button\"" w495 {
                              tunnel: [TRUE w502 TRUE] -> w494
                              frame #0 {
                              }
                              frame #1 {
                                w502 = TRUE
                                n98 = local write "Emergency Stop"(w502) -> ()
                                n99 = Wait (ms)(milliseconds to wait=u32 3000) -> ()  [unwired: 1 out]
                              }
                              frame #2 {
                              }
                            }
                          }
                          frame #1 {
                          }
                        }
                        n100 = case shown="1" w459 {
                          tunnel: w460 -> [_ w472 w473 w474 w475 w476 w477 w478 w479 w480 w481 w482 w483 w484 w485 w486 w487 w488 w489 w490 w491 w492 w493]
                          frame #0 {
                            (unwired) TRUE
                          }
                          frame #1 {
                            n101 = local write "Site 1"(w472) -> ()
                          }
                          frame #2 {
                            n102 = local write "Site 2"(w473) -> ()
                          }
                          frame #3 {
                            n103 = local write "Site 3"(w474) -> ()
                          }
                          frame #4 {
                            n104 = local write "Site 4"(w475) -> ()
                          }
                          frame #5 {
                            n105 = local write "Site 5"(w476) -> ()
                          }
                          frame #6 {
                            n106 = local write "Site 6"(w477) -> ()
                          }
                          frame #7 {
                            n107 = local write "Site 7"(w478) -> ()
                          }
                          frame #8 {
                            n108 = local write "Site 8"(w479) -> ()
                          }
                          frame #9 {
                            n109 = local write "Site 9"(w480) -> ()
                          }
                          frame #10 {
                            n110 = local write "Site 10"(w481) -> ()
                          }
                          frame #11 {
                            n111 = local write "Site 11"(w482) -> ()
                          }
                          frame #12 {
                            n112 = local write "Site 12"(w483) -> ()
                          }
                          frame #13 {
                            n113 = local write "Site 13"(w484) -> ()
                          }
                          frame #14 {
                            n114 = local write "Site 14"(w485) -> ()
                          }
                          frame #15 {
                            n115 = local write "Site 15"(w486) -> ()
                          }
                          frame #16 {
                            n116 = local write "Site 16"(w487) -> ()
                          }
                          frame #17 {
                            n117 = local write "Site 17"(w488) -> ()
                          }
                          frame #18 {
                            n118 = local write "Site 18"(w489) -> ()
                          }
                          frame #19 {
                            n119 = local write "Site 19"(w490) -> ()
                          }
                          frame #20 {
                            n120 = local write "Site 20"(w491) -> ()
                          }
                          frame #21 {
                            n121 = local write "Site 21"(w492) -> ()
                          }
                          frame #22 {
                            n122 = local write "Site 22"(w493) -> ()
                          }
                        }
                      }
                    }
                  }
                }
              }
              frame #1 {
                n123 = local write "Site Number"(w506) -> ()
                "Contact Check Result" <- "Skipped"
              }
            }
          }
          frame #2 {
            n124 = Not(x=w517) -> (.not. x?=w516:bool)
            n125 = Compound Arithmetic op=OR(w518, w516, w515) -> (w514:bool)
            n126 = case shown="False" w514 {
              tunnel: w540 -> [w638 _]
              tunnel: w539 -> [w637 _]
              tunnel: w538 -> [w636 w907]
              tunnel: w537 -> [w635 w908]
              tunnel: [w634 w908] -> w536
              tunnel: [w633 w907] -> w535
              tunnel: [w632 w905] -> w534
              tunnel: [w631 w905] -> w533
              tunnel: w532 -> [w630 w904]
              tunnel: [w629 w904] -> w531
              tunnel: w530 -> [w628 _]
              tunnel: w529 -> [w561 _]
              tunnel: [w627 w905] -> w528
              tunnel: w527 -> [w626 _]
              tunnel: w526 -> [w625 _]
              tunnel: w525 -> [w624 _]
              tunnel: [w623 0] -> w524
              tunnel: w523 -> [w622 w903]
              tunnel: [w621 w903] -> w522
              tunnel: w521 -> [w607 _]
              tunnel: w520 -> [w606 _]
              tunnel: w519 -> [w604 _]
              tunnel: w513 -> [w560 _]
              frame #0 {
                (unwired) FALSE
                # "Read \nCurrent"
                # "Set Voltage"
                n127 = flat-sequence {
                  tunnel: [w648] -> w619
                  tunnel: [w647] -> w618
                  tunnel: [w652] -> w617
                  tunnel: [w651] -> w616
                  tunnel: [w650] -> w615
                  tunnel: [w644] -> w614
                  tunnel: w636 -> [w649]
                  tunnel: w635 -> [w647]
                  tunnel: w625 -> [w652]
                  tunnel: w624 -> [w651]
                  tunnel: w622 -> [w650]
                  tunnel: w638 -> [w676]
                  tunnel: w637 -> [w675]
                  tunnel: w605 -> [w671]
                  tunnel: w630 -> [w668]
                  tunnel: w628 -> [w666]
                  tunnel: w561 -> [w665]
                  tunnel: w626 -> [w663]
                  tunnel: w619 -> [w674]
                  tunnel: w618 -> [w657]
                  tunnel: w617 -> [w662]
                  tunnel: w616 -> [w661]
                  tunnel: w615 -> [w659]
                  tunnel: w614 -> [w655]
                  tunnel: [w673] -> w559
                  tunnel: [w672] -> w557
                  tunnel: [w670] -> w555
                  tunnel: [w669] -> w553
                  tunnel: [w667] -> w551
                  tunnel: [w664] -> w549
                  tunnel: [w660] -> w547
                  tunnel: [w658] -> w545
                  tunnel: [w654] -> w543
                  tunnel: [w653] -> w541
                  tunnel: w559 -> [w869]
                  tunnel: [w869] -> w558
                  tunnel: w557 -> [w868]
                  tunnel: [w868] -> w556
                  tunnel: w555 -> [w867]
                  tunnel: [w867] -> w554
                  tunnel: w553 -> [w866]
                  tunnel: [w866] -> w552
                  tunnel: w551 -> [w865]
                  tunnel: [w865] -> w550
                  tunnel: w549 -> [w864]
                  tunnel: [w864] -> w548
                  tunnel: w547 -> [w863]
                  tunnel: [w863] -> w546
                  tunnel: w545 -> [w862]
                  tunnel: [w862] -> w544
                  tunnel: w543 -> [w861]
                  tunnel: [w861] -> w542
                  tunnel: w541 -> [w860]
                  tunnel: [w894] -> w621
                  tunnel: [w895] -> w623
                  tunnel: [w896] -> w627
                  tunnel: [w897] -> w629
                  tunnel: [w898] -> w631
                  tunnel: [w899] -> w632
                  tunnel: [w900] -> w633
                  tunnel: [w901] -> w634
                  tunnel: w558 -> [w901]
                  tunnel: w556 -> [w900]
                  tunnel: w554 -> [w899]
                  tunnel: w552 -> [w898]
                  tunnel: w550 -> [w897]
                  tunnel: w548 -> [w896]
                  tunnel: w546 -> [w895]
                  tunnel: w544 -> [w894]
                  tunnel: w542 -> [w893]
                  tunnel: w604 -> [w892]
                  tunnel: [w872] -> w597
                  tunnel: [w870] -> w563
                  frame #0 {
                    n128 = local read "Bias Polarity"() -> (w644:dbl)
                    n129 = call "Keith 237 Operate/Standby.vi"("source"=TRUE, "error in"=w649, "GPIB address"=w647) -> ("error out"=w648:T2)
                    n130 = Wait (ms)(milliseconds to wait=u32 1000) -> ()  [unwired: 1 out]
                    n131 = local write "Status"("Starting IV Sensor Scan" ("Status")) -> ()
                  }
                  frame #1 {
                    w656 = TRUE
                    n132 = while {
                      tunnel: w675 -> [w770]
                      tunnel: [w691] -> w673
                      tunnel: w676 -> [w764]
                      shift-right: [w767] -> w672
                      shift-left: w674 -> [w765]
                      tunnel: w671 -> [w761]
                      tunnel: [w760] -> w664
                      tunnel: [w759] -> w670
                      tunnel: [w753] -> w669
                      tunnel: w668 -> [w757]
                      tunnel: [w756] -> w667
                      tunnel: w666 -> [w755]
                      tunnel: w665 -> [w754]
                      tunnel: [w740] -> w660
                      tunnel: w663 -> [w739]
                      tunnel: w662 -> [w737]
                      tunnel: w661 -> [w736]
                      tunnel: w659 -> [w707]
                      tunnel: [w706] -> w658
                      shift-right: [w679] -> _
                      shift-left: w656 -> [w697]
                      shift-left: w656 -> [w699]
                      shift-left: w656 -> [w698]
                      tunnel: w657 -> [w690]
                      shift-left: w656 -> [w684]
                      shift-left: w656 -> [w683]
                      tunnel: w655 -> [w682]
                      tunnel: [w681] -> w654 mode=indexing
                      tunnel: [w677] -> w653
                      i -> [w758]
                      stop <- w747 continue-if-true
                      # "Change Bias Polarity\n+1 Chuck Bias\n-1  Pad bias"
                      # "Loop timing"
                      # "Plot Current"
                      n133 = Build Array(w697, w698, w699, w684, w683) -> (w696:bool[])
                      n134 = case shown="True" "Halt IV" {
                        selector: "Halt IV" -> [_ w776]
                        tunnel: [FALSE ("source") w779] -> w749
                        tunnel: w687 -> [_ w774]
                        frame #0 {
                        }
                        frame #1 {
                          n135 = flat-sequence {
                            tunnel: w776 -> [w782]
                            tunnel: [w782] -> w777
                            tunnel: w774 -> [w780]
                            tunnel: [w780] -> w772
                            tunnel: [w784] -> w778
                            tunnel: w777 -> [w785]
                            tunnel: [w783] -> w773
                            tunnel: w772 -> [w783]
                            tunnel: w778 -> [w788]
                            tunnel: [w788] -> w775
                            tunnel: w773 -> [w786]
                            tunnel: [w790] -> w779
                            tunnel: w775 -> [w790]
                            frame #0 {
                              n136 = call "Keith 237 Operate/Standby.vi"("source"=FALSE, "GPIB address"=w780) -> ()  [unwired: 1 in, 1 out]
                            }
                            frame #1 {
                              n137 = call "Prompt User for Input"("Enable"=w785) -> ("Yes"=w784:bool)  [unwired: 17 in, 1 out]
                            }
                            frame #2 {
                              n138 = call "Keith 237 Operate/Standby.vi"("source"=TRUE, "GPIB address"=w786) -> ()  [unwired: 1 in, 1 out]
                            }
                            frame #3 {
                              n139 = Wait (ms)(milliseconds to wait=750) -> ()  [unwired: 1 out]
                            }
                          }
                        }
                      }
                      n140 = Multiply(x=w764, y=w758) -> (x*y=w751:i32)
                      n141 = Multiply(x=w682, y=w751) -> (x*y=w738:dbl)
                      n142 = Equal To 0?(x=w758) -> (x = 0?=w745:bool)
                      n143 = flat-sequence {
                        tunnel: w736 -> [w794]
                        tunnel: w737 -> [w795]
                        tunnel: w765 -> [w796]
                        tunnel: [w796] -> w729
                        tunnel: [w795] -> w728
                        tunnel: [w794] -> w727
                        tunnel: [w793] -> w712
                        tunnel: w707 -> [w792]
                        tunnel: w690 -> [w791]
                        tunnel: [w791] -> w689
                        tunnel: w738 -> [w801]
                        tunnel: [w803] -> w735
                        tunnel: [w800] -> w734
                        tunnel: [w799] -> w733
                        tunnel: w729 -> [w802]
                        tunnel: w728 -> [w800]
                        tunnel: w727 -> [w799]
                        tunnel: [w798] -> w713
                        tunnel: w712 -> [w798]
                        tunnel: [w797] -> w692
                        tunnel: w689 -> [w797]
                        tunnel: w735 -> [w809]
                        tunnel: w734 -> [w808]
                        tunnel: w733 -> [w807]
                        tunnel: [w809] -> w732
                        tunnel: [w808] -> w731
                        tunnel: [w807] -> w730
                        tunnel: w713 -> [w806]
                        tunnel: [w805] -> w710
                        tunnel: [w804] -> w693
                        tunnel: w692 -> [w804]
                        tunnel: w732 -> [w812]
                        tunnel: w731 -> [w815]
                        tunnel: w730 -> [w814]
                        tunnel: [w811] -> w726
                        tunnel: [w815] -> w725
                        tunnel: [w814] -> w724
                        tunnel: [w813] -> w711
                        tunnel: w710 -> [w813]
                        tunnel: [w810] -> w694
                        tunnel: w693 -> [w810]
                        tunnel: w726 -> [w821]
                        tunnel: w725 -> [w820]
                        tunnel: w724 -> [w819]
                        tunnel: [w821] -> w723
                        tunnel: [w820] -> w722
                        tunnel: [w819] -> w721
                        tunnel: w711 -> [w818]
                        tunnel: [w817] -> w708
                        tunnel: [w816] -> w695
                        tunnel: w694 -> [w816]
                        tunnel: w723 -> [w832]
                        tunnel: w722 -> [w829]
                        tunnel: w721 -> [w828]
                        tunnel: [w822] -> w720
                        tunnel: [w824] -> w719
                        tunnel: [w823] -> w718
                        tunnel: [w827] -> w715
                        tunnel: [w826] -> w709
                        tunnel: w708 -> [w826]
                        tunnel: w695 -> [w825]
                        tunnel: [w825] -> w691
                        tunnel: [w825] -> w688
                        tunnel: [w822] -> w680
                        tunnel: w720 -> [w839]
                        tunnel: w719 -> [w838]
                        tunnel: w718 -> [w837]
                        tunnel: [w839] -> w717
                        tunnel: [w838] -> w716
                        tunnel: [w837] -> w685
                        tunnel: [w836] -> w714
                        tunnel: w715 -> [w836]
                        tunnel: w709 -> [w835]
                        tunnel: [w834] -> w706
                        tunnel: w688 -> [w833]
                        tunnel: [w833] -> w687
                        frame #0 {
                          n144 = call <vilib>:"Acquire Semaphore.vi"("semaphore"=w792) -> ("semaphore out"=w793:T1)  [unwired: 4 in, 2 out]
                        }
                        frame #1 {
                          n145 = call "Kei237_Set_Volt.vi"("Voltage"=w801, "error in"=w802, "GPIB"=w797) -> ("error out"=w803:errorcluster)
                        }
                        frame #2 {
                          n146 = call <vilib>:"Release Semaphore.vi"("semaphore"=w806) -> ("semaphore out"=w805:T1)  [unwired: 5 in, 1 out]
                        }
                        frame #3 {
                          n147 = call "Time Delay4"("error in (no error)"=w812) -> ("error out"=w811:errorcluster)  [unwired: 10 in]
                        }
                        frame #4 {
                          n148 = call <vilib>:"Acquire Semaphore.vi"("semaphore"=w818) -> ("semaphore out"=w817:T1)  [unwired: 4 in, 2 out]
                        }
                        frame #5 {
                          # "14"
                          # "10"
                          n149 = call "K237-read-current-2.vi"("error in"=w832, "GPIB"=w825) -> ("error out"=w831:T2, "Current"=w822:dbl)
                          n150 = call "KE6485 Read.vi"("error in (no error)"=w831, "instrument handle"=w829) -> ("error out"=w830:errorcluster, "reading"=w824:dbl)  [unwired: 7 in, 1 out]
                          n151 = call "KE6485 Read.vi"("error in (no error)"=w830, "instrument handle"=w828) -> ("error out"=w827:errorcluster, "reading"=w823:dbl)  [unwired: 7 in, 1 out]
                        }
                        frame #6 {
                          n152 = call <vilib>:"Release Semaphore.vi"("semaphore"=w835) -> ("semaphore out"=w834:T1)  [unwired: 5 in, 1 out]
                        }
                      }
                      n153 = local write "K237_Bias"(w738) -> ()
                      n154 = local read "voltage \ncompliance cutoff"() -> (w686:dbl)
                      n155 = Absolute Value(x=w680) -> (abs(x)=w678:dbl)
                      n156 = Absolute Value(x=w738) -> (abs(x)=w741:dbl)
                      n157 = Less?(x=w678, y=w686) -> (x < y?=w679:bool)
                      n158 = Not(x=w749) -> (.not. x?=w748:bool)
                      n159 = Wait Until Next ms Multiple(millisecond multiple=u32 1000) -> ()  [unwired: 1 out]
                      n160 = Select(t=w741, s=w739, f=w738) -> (s? t:f=w740:dbl)
                      n161 = Absolute Value(x=w740) -> (abs(x)=w705:dbl)
                      n162 = Absolute Value(x=w770) -> (abs(x)=w746:i32)
                      n163 = Or Array Elements(Boolean array=w696) -> (logical OR=w700:bool)
                      n164 = Less?(x=w705, y=w746) -> (x < y?=w750:bool)
                      n165 = Absolute Value(x=w717) -> (abs(x)=w744:dbl)
                      n166 = Absolute Value(x=w716) -> (abs(x)=w743:dbl)
                      n167 = Absolute Value(x=w685) -> (abs(x)=w742:dbl)
                      n168 = Compound Arithmetic op=AND(w700, w750, w748) -> (w747:bool)
                      n169 = Select(t=w744, s=w739, f=w717) -> (s? t:f=w704:dbl)
                      n170 = Select(t=w743, s=w739, f=w716) -> (s? t:f=w702:dbl)
                      n171 = Select(t=w742, s=w739, f=w685) -> (s? t:f=w703:dbl)
                      n172 = call "Total Current"("error in (no error)"=w714, "Reset"=w745, "Y Input"=w704, "X Input"=w740) -> ("error out"=w767:errorcluster, "XY Graph"=w753:cluster{"Y":dbl[], "Y":dbl[]}[])  [unwired: 1 in, 5 out]
                      "Total Current" <- w753
                      n173 = call "6485 Top"("error in (no error)"=w714, "Reset"=w745, "Y Input"=w702, "X Input"=w740) -> ("error out"=→"error out 5":errorcluster, "XY Graph"=w759:cluster{"Y":dbl[], "Y":dbl[]}[])  [unwired: 1 in, 5 out]
                      "6485 GRD (GPIB 10)" <- w759
                      n174 = call "6485 Bottom"("error in (no error)"=w714, "Reset"=w745, "Y Input"=w703, "X Input"=w740) -> ("error out"=→"error out 4":errorcluster, "XY Graph"=w760:cluster{"Y":dbl[], "Y":dbl[]}[])  [unwired: 1 in, 5 out]
                      "6485 ACTIVE (GPIB 14)" <- w760
                      n175 = Build Array(w740, w704, w703, w702) -> (w681:dbl[])
                      n176 = call-poly <vilib>:"Write To Spreadsheet File.vi"("delimiter (\\t)"="," ("delimiter (\\t)"), "format (%.3f)"="%.3e" ("file format"), "append to file? (new file:F)"=TRUE ("transpose? (no:F)"), "1D data"=w681, "file path (dialog if empty)"=w761) -> ("new file path (Not A Path if cancelled)"=w677:path)  [unwired: 2 in, 1 out]
                      n177 = call "XML_Data.vi"("Data Input Array"=w681, "Data Tag Names Array"=w755, "XML File Path"=w754, "DOM document in"=w757) -> ("DOM document out"=w756:refnum<k20>)  [unwired: 6 in, 1 out]
                    }
                  }
                  frame #2 {
                    n178 = local read "voltage \ncompliance level"() -> (w858:dbl)
                    n179 = local read "Bias Polarity"() -> (w855:dbl)
                    n180 = local read "IV-V-Steps"() -> (w856:i32)
                    n181 = local read "IV-V-Limit"() -> (w857:i32)
                    n182 = local read "Site # IV"() -> (w859:dbl)
                    n183 = Number To Fractional String(number=w859) -> (F-format string=w854:string)  [unwired: 3 in]
                    n184 = Number To Exponential String(number=w858) -> (E-format string=w853:string)  [unwired: 3 in]
                    n185 = Number To Fractional String(number=w855) -> (F-format string=w852:string)  [unwired: 3 in]
                    n186 = Number To Fractional String(number=w856) -> (F-format string=w851:string)  [unwired: 3 in]
                    n187 = Number To Fractional String(number=w857) -> (F-format string=w850:string)  [unwired: 3 in]
                    n188 = Build Array("K237 Parameters" ("string"), "Site Number" ("string"), "Voltage Compliance Level" ("string"), "Bias Polarity" ("string"), "Voltage Steps" ("string"), "Voltage Limit" ("string")) -> (w842:string[])
                    n189 = Build Array("", w854, w853, w852, w851, w850) -> (w841:string[])
                    n190 = Build Array(w842, w841) -> (w840:string[][])
                    n191 = call "Manual CV paramter_append.vi"("Array"=w840, "Path"=w860) -> ()  [unwired: 9 in, 1 out]
                  }
                  frame #3 {
                    n192 = call "IV_Sensor_Check.vi"("Data"=w893, "Titles"=w892) -> ("Boolean Pass/Fail Array"=w870:bool[], "Test Check Names"=w872:string[])  [unwired: 8 in]
                    n193 = Index Array(array=w872, index=0) -> (element=w891:string)
                    n194 = Index Array(array=w872, index=1) -> (element=w885:string)
                    n195 = Index Array(array=w872, index=2) -> (element=w884:string)
                    n196 = Index Array(array=w872, index=3) -> (element=w883:string)
                    n197 = Index Array(array=w872, index=4) -> (element=w882:string)
                    n198 = property on="Boolean" class="Bool (strict)"("Caption.Text"=w891) -> ()  [unwired: 2 in, 2 out]
                    n199 = property on="Boolean 2" class="Bool (strict)"("Caption.Text"=w885) -> ()  [unwired: 2 in, 2 out]
                    n200 = property on="Boolean 3" class="Bool (strict)"("Caption.Text"=w884) -> ()  [unwired: 2 in, 2 out]
                    n201 = property on="Boolean 4" class="Bool (strict)"("Caption.Text"=w883) -> ()  [unwired: 2 in, 2 out]
                    n202 = property on="Boolean 5" class="Bool (strict)"("Caption.Text"=w882) -> ()  [unwired: 2 in, 2 out]
                    n203 = Index Array(array=w870, index=0) -> (element=w876:bool)
                    n204 = Index Array(array=w870, index=1) -> (element=w874:bool)
                    n205 = Index Array(array=w870, index=2) -> (element=w871:bool)
                    n206 = Index Array(array=w870, index=3) -> (element=w873:bool)
                    n207 = Index Array(array=w870, index=4) -> (element=w875:bool)
                    n208 = local write "Boolean"(w876) -> ()
                    n209 = local write "Boolean 2"(w874) -> ()
                    n210 = local write "Boolean 3"(w871) -> ()
                    n211 = local write "Boolean 4"(w873) -> ()
                    n212 = local write "Boolean 5"(w875) -> ()
                  }
                }
                n213 = Open/Create/Replace File(file path (use dialog)=w606, operation (0:open)=T5."replace or create", access (0:read/write)=enum16{"read/write", "read-only", "write-only"}."read/write") -> (refnum out=w611:refnum<file>)  [unwired: 1 in, 4 out]
                n214 = Refnum to Path(1:w611) -> (0:w610:path)
                n215 = call-poly <vilib>:"Write To Spreadsheet File.vi"("delimiter (\\t)"="," ("delimiter (\\t)"), "append to file? (new file:F)"=FALSE, "2D data"=w607, "file path (dialog if empty)"=w610) -> ("new file path (Not A Path if cancelled)"=w605:path)  [unwired: 4 in]
                n216 = local write "Running Conditional"(TRUE) -> ()
                n217 = for {
                  tunnel: w563 -> [w642] mode=indexing
                  tunnel: [w639] -> w562 mode=indexing
                  n218 = Select(t="Passed" ("element"), s=w642, f="Failed" ("element")) -> (s? t:f=w639:string)
                }
                n219 = local read "File Name"() -> (w568:string)
                n220 = Concatenate Strings(w568, "_Check.csv" ("string")) -> (w569:string)
                n221 = Strip Path(path=w560) -> (stripped path=w572:path)  [unwired: 1 out]
                n222 = Index Array(array=w597, index=0) -> (element=w596:string)
                n223 = Index Array(array=w597, index=1) -> (element=w595:string)
                n224 = Index Array(array=w597, index=2) -> (element=w594:string)
                n225 = Index Array(array=w597, index=3) -> (element=w593:string)
                n226 = Index Array(array=w597, index=4) -> (element=w592:string)
                n227 = property on="Tab Control 2" class="TabCtl (strict)"("Visible"=TRUE) -> ()  [unwired: 2 in, 2 out]
                n228 = Index Array(array=w562, index=0) -> (element=w586:string)
                n229 = Index Array(array=w562, index=1) -> (element=w585:string)
                n230 = Index Array(array=w562, index=2) -> (element=w584:string)
                n231 = Index Array(array=w562, index=3) -> (element=w583:string)
                n232 = Index Array(array=w562, index=4) -> (element=w582:string)
                n233 = Build Path(base path=w572, name or relative path=w569) -> (appended path=w571:path)
                n234 = Build Array(w596, w595, w594, w593, w592) -> (w581:string[])
                n235 = Build Array(w586, w585, w584, w583, w582) -> (w580:string[])
                n236 = Build Array(w568, "Passed/Failed" ("element")) -> (w565:string[])
                n237 = Build Array(w581, w580) -> (w579:string[][])
                n238 = Transpose 2D Array(2D array=w579) -> (transposed array=w564:string[][])
                n239 = Open/Create/Replace File(file path (use dialog)=w571, operation (0:open)=T5."replace or create", access (0:read/write)=enum16{"read/write", "read-only", "write-only"}."read/write") -> (refnum out=w577:refnum<file>)  [unwired: 1 in, 4 out]
                n240 = Refnum to Path(1:w577) -> (0:w574:path)
                n241 = Build Array (concatenate)(w565, w564) -> (w566:string[][])
                n242 = call-poly <vilib>:"Write To Spreadsheet File.vi"("delimiter (\\t)"="," ("delimiter (\\t)"), "append to file? (new file:F)"=FALSE, "2D data"=w566, "file path (dialog if empty)"=w574) -> ()  [unwired: 4 in, 1 out]
              }
              frame #1 {
                w902 = FALSE ("Boolean")
                w905 = cluster{"Y":dbl[], "Y":dbl[]}[] [] ("XY Graph")
                n243 = local write "Boolean"(w902) -> ()
                n244 = local write "Boolean 2"(w902) -> ()
                n245 = local write "Boolean 3"(w902) -> ()
                n246 = local write "Boolean 4"(w902) -> ()
                n247 = local write "Boolean 5"(w902) -> ()
              }
            }
            n248 = call-poly <vilib>:"Close.vi"("node"=w531) -> ()  [unwired: 8 in, 1 out]
          }
          frame #3 {
            w909 = FALSE
            n249 = case shown="True" w909 {
              tunnel: w914 -> [w919 w924]
              tunnel: [w919 w923] -> w913
              tunnel: [w918 w922] -> w912
              tunnel: w911 -> [_ w921]
              tunnel: w910 -> [w918 w920]
              frame #0 {
              }
              frame #1 {
                n250 = while {
                  tunnel: [w940] -> w922
                  tunnel: w924 -> [w934]
                  tunnel: [w934] -> w923
                  tunnel: w921 -> [w928]
                  tunnel: w920 -> [w925]
                  i -> [w939]
                  stop <- w936 continue-if-true
                  n251 = Multiply(x=400, y=w939) -> (x*y=w931:i32)
                  n252 = Sign(1:w928) -> (0:w933:dbl)
                  n253 = Subtract(x=w928, y=w931) -> (x-y=w930:dbl)
                  n254 = Add(x=w928, y=w931) -> (x+y=w929:dbl)
                  n255 = Greater Than 0?(x=w933) -> (x > 0?=w932:bool)
                  n256 = Select(t=w930, s=w932, f=w929) -> (s? t:f=w926:dbl)
                  n257 = Absolute Value(x=w926) -> (abs(x)=w927:dbl)
                  n258 = local write "K237_Bias"(w926) -> ()
                  n259 = call "Time Delay"("error in (no error)"=w925) -> ("error out"=w935:errorcluster)  [unwired: 10 in]
                  n260 = Greater?(x=w927, y=400) -> (0:w936:bool)
                  n261 = call "Kei237_Set_Volt.vi"("Voltage"=w926, "error in"=w935, "GPIB"=w934) -> ("error out"=w940:errorcluster)
                }
              }
            }
            n262 = local write "Running Conditional"(w909) -> ()
            n263 = local write "Running?"(w909) -> ()
          }
          frame #4 {
            n264 = Wait (ms)(milliseconds to wait=250) -> ()  [unwired: 1 out]
          }
          frame #5 {
            w947 = TRUE ("append to file? (new file:F)")
            w988 = 0
            n265 = local read "Site Number"() -> (w958:i32)
            n266 = In Range and Coerce(upper limit=3, x=w1001, lower limit=0) -> (In Range?=w977:bool)  [unwired: 1 out]
            n267 = case shown="False" w977 {
              tunnel: [w1128 w1140] -> w1004
              tunnel: w1001 -> [w1127 _]
              frame #0 {
                n268 = In Range and Coerce(upper limit=11, x=w1127, lower limit=4) -> (In Range?=w1129:bool)  [unwired: 1 out]
                n269 = case shown="False" w1129 {
                  tunnel: [w1136 w1139] -> w1128
                  tunnel: w1127 -> [w1133 _]
                  frame #0 {
                    n270 = In Range and Coerce(upper limit=17, x=w1133, lower limit=12) -> (In Range?=w1132:bool)  [unwired: 1 out]
                    n271 = case shown="False" w1132 {
                      tunnel: [w1137 w1138] -> w1136
                      frame #0 {
                        w1137 = 3
                        n272 = property on="Archive" class="TabCtl (strict)"("Value"=w1137) -> ()  [unwired: 2 in, 2 out]
                      }
                      frame #1 {
                        w1138 = 1
                        n273 = property on="Archive" class="TabCtl (strict)"("Value"=w1138) -> ()  [unwired: 2 in, 2 out]
                      }
                    }
                  }
                  frame #1 {
                    w1139 = 2
                    n274 = property on="Archive" class="TabCtl (strict)"("Value"=w1139) -> ()  [unwired: 2 in, 2 out]
                  }
                }
              }
              frame #1 {
                w1140 = 0
                n275 = property on="Archive" class="TabCtl (strict)"("Value"=w1140) -> ()  [unwired: 2 in, 2 out]
              }
            }
            n276 = local write "Status"("IV Sensor Scan Finished" ("Status")) -> ()
            n277 = case shown="1, Default" w958 {
              tunnel: ["D_BL_" "D_TL_" "D_TR_" "D_BR_" "L_TT_" "L_FL_" "L_LL_" "L_CL_" "L_CR_" "L_RR_" "L_FR_" "L_BB_" "S_TL_" "S_TR_" "S_CL_" "S_CR_" "S_BL_" "S_BR_" "A_TL_" "A_TR_" "A_BL_" "A_BR_"] -> w957
              tunnel: ["Diode" "Diode" "Diode" "Diode" w1021 w1027 w1033 w1039 w1045 w1051 w1057 w1063 w1069 w1075 w1081 w1087 w1093 w1099 w1105 w1112 w1118 w1124] -> _
              tunnel: ["D1" "D2" "D3" "D4" "L5-2x8" "L6-2x8" "L7-2x8" "L8-2x8" "L9-2x8" "L10-2x8" "L11-2x8" "L12-2x8" "S13-1x1" "S14-1x1" "S15-1x1" "S16-1x1" "S17-1x1" "S18-1x1" "SE19" "SE20" "SE21" "SE22"] -> _
              frame #0 {
              }
              frame #1 {
              }
              frame #2 {
              }
              frame #3 {
              }
              frame #4 {
                n278 = call <vilib>:"Space Constant.vi"() -> ("String"=w1023:string)
                n279 = Concatenate Strings("2x8", w1023, "X") -> (w1021:string)
              }
              frame #5 {
                n280 = call <vilib>:"Space Constant.vi"() -> ("String"=w1029:string)
                n281 = Concatenate Strings("2x8", w1029, "FMM") -> (w1027:string)
              }
              frame #6 {
                n282 = call <vilib>:"Space Constant.vi"() -> ("String"=w1035:string)
                n283 = Concatenate Strings("2x8", w1035, "FMM") -> (w1033:string)
              }
              frame #7 {
                n284 = call <vilib>:"Space Constant.vi"() -> ("String"=w1041:string)
                n285 = Concatenate Strings("2x8", w1041, "Close") -> (w1039:string)
              }
              frame #8 {
                n286 = call <vilib>:"Space Constant.vi"() -> ("String"=w1047:string)
                n287 = Concatenate Strings("2x8", w1047, "X") -> (w1045:string)
              }
              frame #9 {
                n288 = call <vilib>:"Space Constant.vi"() -> ("String"=w1053:string)
                n289 = Concatenate Strings("2x8", w1053, "FM") -> (w1051:string)
              }
              frame #10 {
                n290 = call <vilib>:"Space Constant.vi"() -> ("String"=w1059:string)
                n291 = Concatenate Strings("2x8", w1059, "FM") -> (w1057:string)
              }
              frame #11 {
                n292 = call <vilib>:"Space Constant.vi"() -> ("String"=w1065:string)
                n293 = Concatenate Strings("2x8", w1065, "Close") -> (w1063:string)
              }
              frame #12 {
                n294 = call <vilib>:"Space Constant.vi"() -> ("String"=w1071:string)
                n295 = Concatenate Strings("1x1", w1071, "FMM") -> (w1069:string)
              }
              frame #13 {
                n296 = call <vilib>:"Space Constant.vi"() -> ("String"=w1077:string)
                n297 = Concatenate Strings("1x1", w1077, "FMM") -> (w1075:string)
              }
              frame #14 {
                n298 = call <vilib>:"Space Constant.vi"() -> ("String"=w1083:string)
                n299 = Concatenate Strings("1x1", w1083, "Close") -> (w1081:string)
              }
              frame #15 {
                n300 = call <vilib>:"Space Constant.vi"() -> ("String"=w1089:string)
                n301 = Concatenate Strings("1x1", w1089, "FM") -> (w1087:string)
              }
              frame #16 {
                n302 = call <vilib>:"Space Constant.vi"() -> ("String"=w1095:string)
                n303 = Concatenate Strings("1x1", w1095, "X") -> (w1093:string)
              }
              frame #17 {
                n304 = call <vilib>:"Space Constant.vi"() -> ("String"=w1101:string)
                n305 = Concatenate Strings("1x1", w1101, "FMM") -> (w1099:string)
              }
              frame #18 {
                n306 = call <vilib>:"Space Constant.vi"() -> ("String"=w1107:string)
                n307 = Concatenate Strings("Slim-Edge", w1107, "FMM_S3") -> (w1105:string)
              }
              frame #19 {
                n308 = call <vilib>:"Space Constant.vi"() -> ("String"=w1113:string)
                n309 = Concatenate Strings("Slim-Edge", w1113, "FMM_S3") -> (w1112:string)
              }
              frame #20 {
                n310 = call <vilib>:"Space Constant.vi"() -> ("String"=w1119:string)
                n311 = Concatenate Strings("Slim-Edge", w1119, "FMM_S3") -> (w1118:string)
              }
              frame #21 {
                n312 = call <vilib>:"Space Constant.vi"() -> ("String"=w1125:string)
                n313 = Concatenate Strings("Slim-Edge", w1125, "FMM_S3") -> (w1124:string)
              }
            }
            n314 = call "Kei237_Set_Volt.vi"("Voltage"=w988, "error in"=w1006, "GPIB"=w969) -> ("error out"=w970:errorcluster)
            n315 = local write "K237_Bias"(w988) -> ()
            n316 = local read "Wafer Number"() -> (w955:string)
            n317 = Unbundle(w987) -> (w986:cluster{"Y":dbl[], "Y":dbl[]}[], w985:cluster{"Y":dbl[], "Y":dbl[]}[], w978:cluster{"Y":dbl[], "Y":dbl[]}[], w984:cluster{"Y":dbl[], "Y":dbl[]}[], w983:cluster{"Y":dbl[], "Y":dbl[]}[], w982:cluster{"Y":dbl[], "Y":dbl[]}[], w981:cluster{"Y":dbl[], "Y":dbl[]}[], w980:cluster{"Y":dbl[], "Y":dbl[]}[], w979:cluster{"Y":dbl[], "Y":dbl[]}[], w974:cluster{"Y":dbl[], "Y":dbl[]}[], w975:cluster{"Y":dbl[], "Y":dbl[]}[], w976:cluster{"Y":dbl[], "Y":dbl[]}[])
            n318 = call "Keith 237 Operate/Standby.vi"("source"=FALSE, "error in"=w970, "GPIB address"=w969) -> ("error out"=w967:T2)
            n319 = Concatenate Strings("W" ("string"), w957, w955) -> (w953:string)
            n320 = case shown="0, Default" w1004 {
              tunnel: w1000 -> [w1158 w1176 w1194 w1212]
              tunnel: w999 -> [w1157 w1175 w1193 w1211]
              tunnel: w998 -> [w1156 w1174 w1192 w1210]
              tunnel: [w1146 w1172 w1189 w1209] -> w997
              tunnel: [w1144 w1170 w1190 w1208] -> w996
              tunnel: [w1145 w1171 w1191 w1207] -> w995
              tunnel: w986 -> [w1155 w1172 w1189 w1209]
              tunnel: w985 -> [w1154 w1170 w1190 w1208]
              tunnel: w978 -> [w1153 w1171 w1191 w1207]
              tunnel: [w1152 w1169 w1188 w1206] -> w994
              tunnel: [w1147 w1162 w1182 w1201] -> w993
              tunnel: [w1149 w1166 w1187 w1205] -> w992
              tunnel: w984 -> [w1152 w1173 w1188 w1206]
              tunnel: w979 -> [w1147 w1162 w1184 w1201]
              tunnel: w983 -> [w1149 w1168 w1187 w1205]
              tunnel: [w1151 w1165 w1186 w1204] -> w991
              tunnel: [w1148 w1164 w1180 w1203] -> w990
              tunnel: [w1150 w1163 w1181 w1202] -> w989
              tunnel: w982 -> [w1151 w1167 w1186 w1204]
              tunnel: w981 -> [w1148 w1164 w1185 w1203]
              tunnel: w980 -> [w1150 w1163 w1183 w1202]
              tunnel: w976 -> [w1141 w1159 w1177 w1199]
              tunnel: w975 -> [w1142 w1160 w1178 w1198]
              tunnel: w974 -> [w1143 w1161 w1179 w1200]
              tunnel: [w1143 w1161 w1179 w1197] -> w973
              tunnel: [w1142 w1160 w1178 w1196] -> w972
              tunnel: [w1141 w1159 w1177 w1195] -> w971
              frame #0 {
                # "Diodes"
                n321 = Insert Into Array(array=w1155, new element=w1158) -> (w1146:cluster{"Y":dbl[], "Y":dbl[]}[])  [unwired: 1 in]
                "Diode ACTIVE Archive" <- w1146
                n322 = Insert Into Array(array=w1154, new element=w1157) -> (w1144:cluster{"Y":dbl[], "Y":dbl[]}[])  [unwired: 1 in]
                "Diode GRD Archive" <- w1144
                n323 = Insert Into Array(array=w1153, new element=w1156) -> (w1145:cluster{"Y":dbl[], "Y":dbl[]}[])  [unwired: 1 in]
                "Diode Total Current Archive" <- w1145
              }
              frame #1 {
                # "Single Chips"
                n324 = Insert Into Array(array=w1173, new element=w1176) -> (w1169:cluster{"Y":dbl[], "Y":dbl[]}[])  [unwired: 1 in]
                "Single Chip ACTIVE Archive" <- w1169
                n325 = Insert Into Array(array=w1168, new element=w1175) -> (w1166:cluster{"Y":dbl[], "Y":dbl[]}[])  [unwired: 1 in]
                "Single Chip GRD Archive" <- w1166
                n326 = Insert Into Array(array=w1167, new element=w1174) -> (w1165:cluster{"Y":dbl[], "Y":dbl[]}[])  [unwired: 1 in]
                "Single Chip Total Current Archive" <- w1165
              }
              frame #2 {
                # "2x8s"
                n327 = Insert Into Array(array=w1185, new element=w1194) -> (w1180:cluster{"Y":dbl[], "Y":dbl[]}[])  [unwired: 1 in]
                "2x8 ACTIVE Archive" <- w1180
                n328 = Insert Into Array(array=w1183, new element=w1193) -> (w1181:cluster{"Y":dbl[], "Y":dbl[]}[])  [unwired: 1 in]
                "2x8 GRD Archive" <- w1181
                n329 = Insert Into Array(array=w1184, new element=w1192) -> (w1182:cluster{"Y":dbl[], "Y":dbl[]}[])  [unwired: 1 in]
                "2x8 Total Current Archive" <- w1182
              }
              frame #3 {
                # "Slim-Edge"
                n330 = Insert Into Array(array=w1200, new element=w1212) -> (w1197:cluster{"Y":dbl[], "Y":dbl[]}[])  [unwired: 1 in]
                "Slim-Edge ACTIVE Archive" <- w1197
                n331 = Insert Into Array(array=w1198, new element=w1211) -> (w1196:cluster{"Y":dbl[], "Y":dbl[]}[])  [unwired: 1 in]
                "Slim-Edge GRD Archive" <- w1196
                n332 = Insert Into Array(array=w1199, new element=w1210) -> (w1195:cluster{"Y":dbl[], "Y":dbl[]}[])  [unwired: 1 in]
                "Slim-Edge Total Current Archive" <- w1195
              }
            }
            n333 = local read "Contact Check Result"() -> (w959:string)
            n334 = Wait Until Next ms Multiple(millisecond multiple=u32 250) -> ()  [unwired: 1 out]
            n335 = local read "Contact Check"() -> (w965:bool)
            n336 = Equal?(x=w959, y="Skipped" ("Contact Check Result")) -> (x = y?=w961:bool)
            n337 = Select(t="Passed", s=w965, f="Failed") -> (s? t:f=w962:string)
            n338 = Select(t=w959, s=w961, f=w962) -> (s? t:f=w954:string)
            n339 = Build Array(w953) -> (w950:string[])
            n340 = Build Array(w954) -> (w949:string[])
            n341 = Build Array(w950, w949) -> (w948:string[][])
            n342 = call-poly <vilib>:"Write To Spreadsheet File.vi"("delimiter (\\t)"="," ("delimiter (\\t)"), "transpose? (no:F)"=w947, "append to file? (new file:F)"=w947, "2D data"=w948, "file path (dialog if empty)"=w951) -> ()  [unwired: 3 in, 1 out]
          }
        }
        n343 = call "Auto_IV_CV_XML_Excell_Label.vi"("Cluster"=w164, "Loop Count"=w165, "IV or CV"=w166) -> ("File Name"=w162:string, "Excell Cell Title"=w161:string[], "XML Data Tags"=w163:string[])  [unwired: 6 in]
        "File Name" <- w162
        n344 = Build Array("Bias", "Total", "Active", "Guardring") -> (w160:string[])
        n345 = Concatenate Strings(w162, "_IV.csv" ("string")) -> (w211:string)
        n346 = Concatenate Strings(w162, "_IV.xml" ("string")) -> (w209:string)
        n347 = Build Array("VOLTAGE_VOLT", "TOT_CURRENT_AMP", "ACTV_CURRENT_AMP", "GRD_CURRENT_AMP") -> (w168:string[])
        n348 = Build Path(base path=w201, name or relative path=w211) -> (appended path=w139:path)
        n349 = Build Path(base path=w140, name or relative path=w209) -> (appended path=w208:path)
        n350 = Build Array(w161, w160) -> (w159:string[][])
        n351 = call "XML_Initilize.vi"("User Input"=w163) -> ("DOM document out"=w217:refnum<k20>)  [unwired: 10 in]
      }
      n352 = call "KE6485 Close.vi"("error in (no error)"=w124, "instrument handle"=refnum<k15> "GPIB0::10::INSTR") -> ("error out"=w127:errorcluster)  [unwired: 9 in]
      n353 = call "KE6485 Close.vi"("error in (no error)"=w127, "instrument handle"=refnum<k15> "GPIB0::14::INSTR") -> ("error out"=w123:errorcluster)  [unwired: 9 in]
      n354 = call "Keith 237 Reset.vi"("GPIB address"=w136, "error in"=w123) -> ("error out"=w128:T2)
    }
    frame #2 {
      n355 = Wait (ms)(milliseconds to wait=u32 500) -> ()  [unwired: 1 out]
    }
    frame #3 {
      n356 = Build Array(16, 10, 14) -> (w1224:i32[])
      n357 = EnableLocal(2:w1220, 3:w1224, 4:0) -> (0:w1219:errorcluster)  [unwired: 1 out]
      n358 = local write "Status"("Full IV Scan Finished" ("Status")) -> ()
    }
    frame #4 {
      # "Ask the operator to\nchange the wires \nfrom IV to CV"
      n359 = call "RE-WIRE  from IV to CV"("Enable"=TRUE) -> ("OK"=w1227:bool)  [unwired: 17 in, 1 out]
      n360 = local read "semaphore"() -> (w1225:T1)
      n361 = Not(x=w1227) -> (.not. x?=w1228:bool)
      n362 = local write "IV or CV"(1 ("IV or CV")) -> ()
      n363 = Stop(stop? (T)=w1228) -> ()
    }
    frame #5 {
      w1233 = u16 5 items=["auto / auto", "1 nA / 1.1 V", "10 nA / 11 V", "100 nA / 110 V", "0.001 mA / 1100 V", "0.01 mA / 1100 V", "0.1 mA / 1100 V", "1 mA / 1100 V", "10 mA / 1100 V", "100 mA / 1100 V"] ("compliance/\nmeasurement range (auto:0)")
      w1248 = 1e-05 ("current \ncompliance level")
      w1244 = u16 5 items=["auto / auto", "1 nA / 1.1 V", "10 nA / 11 V", "100 nA / 110 V", "0.001 mA / 1100 V", "0.01 mA / 1100 V", "0.1 mA / 1100 V", "1 mA / 1100 V", "10 mA / 1100 V", "100 mA / 1100 V"] ("source range\nI source / V source (auto:0)")
      w1249 = u16 0 items=["voltage/current", "current/voltage"] ("source/measure (V/I:0)")
      w1250 = u16 0 items=["DC", "sweep"] ("function (DC:0)")
      w1236 = "16" ("GPIB address")
      w1252 = 1000.0 ("Time Delay mS")
      w1254 = TRUE ("reset")
      w1258 = 0.5  # Voltage Level
      w1259 = 5.0 ("Number of Averages")
      w1260 = 10000.0 ("Frequency")
      w1261 = u16 7 items=["None", "Cs", "Cp", "Ls", "Lp", "Rs", "Rp", "DF", "Q", "Z", "Y", "Phase", "ESR", "Gp", "Xs", "Bp"] ("Secondary Parameter")
      w1262 = u16 2 items=["AUTO", "Cs", "Cp", "Ls", "Lp", "Rs", "Rp", "DF", "Q", "Z", "Y", "Phase", "ESR", "Gp", "Xs", "Bp"] ("Primary Parameter")
      w1263 = u16 0 items=["Voltage", "Current"] ("Signal Type")
      w1264 = u16 0 items=["Measured", "Deviation", "% Deviation", "No Display"] ("Display")
      w1265 = u16 2 items=["Off", "Internal", "External"] ("Bias")
      n364 = DevClear(2:w1238, 3:i16 16 ("address"), 4:0) -> (0:w1240:errorcluster)  [unwired: 1 out]
      n365 = call "Keith 237 Basic Config.vi"("GPIB address"=w1236, "source/measure (V/I:0)"=w1249, "function (DC:0)"=w1250, "source range\nI source / V source (auto:0)"=w1244, "source level"=0.0, "error in"=w1240, "1100 V range (disabled:F)"=TRUE, "current \ncompliance level"=w1248, "compliance/\nmeasurement range (auto:0)"=w1233) -> ("error out"=w1247:T2)  [unwired: 10 in]
      n366 = call "Keith 237 Operate/Standby.vi"("source"=FALSE, "error in"=w1247, "GPIB address"=w1236) -> ("error out"=w1245:T2)
      n367 = local write "Status"("Setting CV Scan Parameters" ("Status")) -> ()
      n368 = call "Keith 237 Send Trigger.vi"("GPIB address"=w1236, "error in"=w1245) -> ("error out"=w1239:T2)
      n369 = call "7000 Series Initialize.vi"("error in (no error)"=w1239, "reset"=w1254, "ID query"=w1254, "instrument descriptor"="GPIB::4") -> ("error out"=w1266:errorcluster, "Identification"=→"QuadTech Status":string, "VISA session"=w1255:refnum<visa-resource-name>)
      n370 = call "7000 Series Configure.vi"("inst handle in"=w1255, "Primary Parameter"=w1262, "Secondary Parameter"=w1261, "Frequency"=w1260, "Number of Averages"=w1259, "error in"=w1266, "Bias"=w1265, "Display"=w1264, "Signal Type"=w1263, "Optional"="CONF:SWE:SWE OFF", "Time Delay mS"=w1252, "Voltage Level"=w1258) -> ("inst handle out"=w1237:refnum<visa-resource-name>, "Identification"=w1256:string, "error out"=w1235:T8)  [unwired: 13 in]
      n371 = local write "QuadTech Status"(w1256) -> ()
      "Frequency" <- w1260
      "Voltage Level" <- w1258
      "Number of Averages" <- w1259
      "Time Delay mS" <- w1252
      "Primary Parameter" <- w1262
      "Auto Compliance" <- w1248
      "Secondary Parameter" <- w1261
    }
    frame #6 {
      n372 = case shown="0, Default" w1269 {
        frame #0 {
          n373 = local read "Auto Compliance"() -> (w1274:dbl)
          n374 = Multiply(x=w1274, y=0.98) -> (x*y=w1273:dbl)
          n375 = local write "Compliance"(w1273) -> ()
        }
        frame #1 {
          n376 = Multiply(x=1e-09, y=0.98) -> (x*y=→"Compliance":dbl)
        }
        frame #2 {
          n377 = Multiply(x=1e-08, y=0.98) -> (x*y=w1279:dbl)
          n378 = local write "Compliance"(w1279) -> ()
        }
        frame #3 {
          n379 = Multiply(x=1e-07, y=0.98) -> (x*y=w1282:dbl)
          n380 = local write "Compliance"(w1282) -> ()
        }
        frame #4 {
          n381 = Multiply(x=1e-06, y=0.98) -> (x*y=w1285:dbl)
          n382 = local write "Compliance"(w1285) -> ()
        }
        frame #5 {
          n383 = Multiply(x=1e-05, y=0.98) -> (x*y=w1289:dbl)
          n384 = local write "Compliance"(w1289) -> ()
        }
        frame #6 {
          n385 = Multiply(x=0.0001, y=0.98) -> (x*y=w1291:dbl)
          n386 = local write "Compliance"(w1291) -> ()
        }
        frame #7 {
          n387 = Multiply(x=0.001, y=0.98) -> (x*y=w1295:dbl)
          n388 = local write "Compliance"(w1295) -> ()
        }
        frame #8 {
          n389 = Multiply(x=0.001, y=0.98) -> (x*y=w1297:dbl)
          n390 = local write "Compliance"(w1297) -> ()
        }
        frame #9 {
          n391 = Multiply(x=0.001, y=0.98) -> (x*y=w1300:dbl)
          n392 = local write "Compliance"(w1300) -> ()
        }
      }
    }
    frame #7 {
      w1317 = u16 0 items=["Off", "Internal", "External"] ("Bias")
      n393 = for {
        N: w1307 -> [_]
        tunnel: w1320 -> [w1386]
        tunnel: w1319 -> [w1385]
        tunnel: [w1355] -> w1315
        tunnel: [w1354] -> w1313
        shift-right: [w1383] -> w1314
        shift-left: w1318 -> [w1384]
        shift-right: [w1380] -> _
        shift-left: _ -> [w1351]
        shift-right: [w1379] -> _
        shift-left: _ -> [w1350]
        shift-right: [w1378] -> _
        shift-left: _ -> [w1349]
        tunnel: w1310 -> [w1363]
        tunnel: w1306 -> [w1347]
        tunnel: w1304 -> [w1327]
        tunnel: w1303 -> [w1321]
        i -> [w1328]
        # "User Input Array\nElement 0: Comment Description (XML_Header)\nElement 1: Serial Number\nElement 2: Kind of Part\nElement 3: User\nElement 4: Extension Table Name\nElement 5: Comment Description (XML_Data_Set)\nElement 6: Name (XML_Header)\nElement 7: Run Name (XML_Header)"
        # "XML Data Tags for CV scan"
        n394 = Increment(x=w1328) -> (x+1=→"Site # CV":i32)
        n395 = local read "IV or CV"() -> (w1329:i32)
        n396 = Bundle(w1351, w1350, w1349) -> (w1348:T9)  [unwired: 1 in]
        n397 = call "Auto_IV_CV_XML_Excell_Label.vi"("Cluster"=w1327, "Loop Count"=w1328, "IV or CV"=w1329) -> ("File Name"=w1325:string, "Excell Cell Title"=w1324:string[], "XML Data Tags"=w1326:string[])  [unwired: 6 in]
        n398 = flat-sequence {
          tunnel: [w1395] -> w1346
          tunnel: w1386 -> [w1395]
          tunnel: [w1394] -> w1345
          tunnel: w1385 -> [w1394]
          tunnel: [w1393] -> w1344
          tunnel: w1384 -> [w1393]
          tunnel: w1328 -> [w1389]
          tunnel: w1347 -> [w1391]
          tunnel: [w1391] -> w1343
          tunnel: [w1390] -> w1342
          tunnel: [w1389] -> w1332
          tunnel: [w1387] -> w1331
          tunnel: [w1442] -> w1377
          tunnel: [w1441] -> w1376
          tunnel: [w1440] -> w1375
          tunnel: [w1433] -> w1374
          tunnel: [w1432] -> w1369
          tunnel: w1368 -> [w1431]
          tunnel: w1362 -> [w1430]
          tunnel: w1359 -> [w1429]
          tunnel: [w1427] -> w1358
          tunnel: w1331 -> [w1422]
          tunnel: w1332 -> [w1424]
          tunnel: w1342 -> [w1421]
          tunnel: w1343 -> [w1426]
          tunnel: w1344 -> [w1443]
          tunnel: w1345 -> [w1440]
          tunnel: w1346 -> [w1444]
          tunnel: w1323 -> [w1420]
          tunnel: w1322 -> [w1419]
          tunnel: w1377 -> [w1787]
          tunnel: [w1787] -> w1373
          tunnel: w1376 -> [w1786]
          tunnel: [w1786] -> w1372
          tunnel: w1375 -> [w1785]
          tunnel: [w1785] -> w1371
          tunnel: w1374 -> [w1760]
          tunnel: [w1759] -> w1370
          tunnel: w1369 -> [w1759]
          tunnel: w1358 -> [w1758]
          tunnel: [w1758] -> w1357
          tunnel: w1373 -> [w1792]
          tunnel: [w1791] -> w1341
          tunnel: w1372 -> [w1795]
          tunnel: [w1795] -> w1339
          tunnel: w1371 -> [w1794]
          tunnel: [w1793] -> w1337
          tunnel: w1370 -> [w1790]
          tunnel: w1357 -> [w1789]
          tunnel: [w1789] -> w1335
          tunnel: w1341 -> [w1823]
          tunnel: [w1823] -> w1340
          tunnel: w1339 -> [w1822]
          tunnel: [w1822] -> w1338
          tunnel: w1337 -> [w1821]
          tunnel: [w1821] -> w1336
          tunnel: w1335 -> [w1820]
          tunnel: [w1820] -> w1334
          tunnel: [w1846] -> w1355
          tunnel: [w1825] -> w1383
          tunnel: w1340 -> [w1845]
          tunnel: w1338 -> [w1846]
          tunnel: w1336 -> [w1827]
          tunnel: w1328 -> [w1829]
          tunnel: [w1838] -> w1380
          tunnel: [w1837] -> w1379
          tunnel: [w1836] -> w1378
          tunnel: w1334 -> [w1834]
          tunnel: [w1827] -> w1354
          tunnel: w1348 -> [w1833]
          frame #0 {
            n399 = Increment(x=w1389) -> (x+1=w1388:i32)
            n400 = case shown="1" w1388 {
              tunnel: [TRUE w1397 w1398 w1399 w1400 w1401 w1402 w1403 w1404 w1405 w1406 w1407 w1408 w1409 w1410 w1411 w1412 w1413 w1414 w1415 w1416 w1417 w1418] -> w1387
              frame #0 {
              }
              frame #1 {
                n401 = local read "Site 1"() -> (w1397:bool)
              }
              frame #2 {
                n402 = local read "Site 2"() -> (w1398:bool)
              }
              frame #3 {
                n403 = local read "Site 3"() -> (w1399:bool)
              }
              frame #4 {
                n404 = local read "Site 4"() -> (w1400:bool)
              }
              frame #5 {
                n405 = local read "Site 5"() -> (w1401:bool)
              }
              frame #6 {
                n406 = local read "Site 6"() -> (w1402:bool)
              }
              frame #7 {
                n407 = local read "Site 7"() -> (w1403:bool)
              }
              frame #8 {
                n408 = local read "Site 8"() -> (w1404:bool)
              }
              frame #9 {
                n409 = local read "Site 9"() -> (w1405:bool)
              }
              frame #10 {
                n410 = local read "Site 10"() -> (w1406:bool)
              }
              frame #11 {
                n411 = local read "Site 11"() -> (w1407:bool)
              }
              frame #12 {
                n412 = local read "Site 12"() -> (w1408:bool)
              }
              frame #13 {
                n413 = local read "Site 13"() -> (w1409:bool)
              }
              frame #14 {
                n414 = local read "Site 14"() -> (w1410:bool)
              }
              frame #15 {
                n415 = local read "Site 15"() -> (w1411:bool)
              }
              frame #16 {
                n416 = local read "Site 16"() -> (w1412:bool)
              }
              frame #17 {
                n417 = local read "Site 17"() -> (w1413:bool)
              }
              frame #18 {
                n418 = local read "Site 18"() -> (w1414:bool)
              }
              frame #19 {
                n419 = local read "Site 19"() -> (w1415:bool)
              }
              frame #20 {
                n420 = local read "Site 20"() -> (w1416:bool)
              }
              frame #21 {
                n421 = local read "Site 21"() -> (w1417:bool)
              }
              frame #22 {
                n422 = local read "Site 22"() -> (w1418:bool)
              }
            }
            n423 = call "Skip Current Subsite2"() -> ("Skip Subsite"=w1390:bool)  [unwired: 18 in, 1 out]
            n424 = Wait (ms)(milliseconds to wait=u32 250) -> ()  [unwired: 1 out]
          }
          frame #1 {
            n425 = Not(x=w1422) -> (.not. x?=w1423:bool)
            n426 = Or(x=w1423, y=w1421) -> (x .or. y?=w1425:bool)
            n427 = case shown="False" w1425 {
              tunnel: "CV-V-Limit" -> [w1492 _]
              tunnel: "CV-V-Steps" -> [w1491 _]
              tunnel: w1444 -> [w1490 w1752]
              tunnel: w1443 -> [w1489 w1751]
              tunnel: [w1488 w1751] -> w1442
              tunnel: [w1487 w1752] -> w1441
              tunnel: w1440 -> [w1486 _]
              tunnel: [w1485 0 ("number")] -> w1436
              tunnel: [w1484 w1747] -> w1433
              tunnel: [w1483 0] -> w1432
              tunnel: w1431 -> [w1482 w1753]
              tunnel: w1430 -> [w1481 _]
              tunnel: w1429 -> [w1480 _]
              tunnel: [w1479 w1753] -> w1428
              tunnel: [w1478 w1754] -> w1427
              tunnel: w1426 -> [w1477 _]
              tunnel: w1424 -> [w1469 _]
              tunnel: w1420 -> [w1449 w1747]
              tunnel: w1419 -> [w1448 _]
              frame #0 {
                n428 = flat-sequence {
                  tunnel: w1477 -> [w1496]
                  tunnel: w1486 -> [w1497]
                  tunnel: w1489 -> [w1498]
                  tunnel: w1490 -> [w1499]
                  tunnel: w1491 -> [w1500]
                  tunnel: w1492 -> [w1501]
                  tunnel: [w1501] -> w1468
                  tunnel: [w1500] -> w1466
                  tunnel: [w1499] -> w1464
                  tunnel: [w1498] -> w1462
                  tunnel: [w1497] -> w1460
                  tunnel: [w1496] -> w1458
                  tunnel: w1469 -> [w1494]
                  tunnel: w1468 -> [w1509]
                  tunnel: [w1509] -> w1467
                  tunnel: w1466 -> [w1508]
                  tunnel: [w1508] -> w1465
                  tunnel: w1464 -> [w1507]
                  tunnel: [w1507] -> w1463
                  tunnel: w1462 -> [w1506]
                  tunnel: [w1506] -> w1461
                  tunnel: w1460 -> [w1505]
                  tunnel: [w1505] -> w1459
                  tunnel: w1458 -> [w1504]
                  tunnel: [w1504] -> w1457
                  tunnel: [w1520] -> w1475
                  tunnel: [w1519] -> w1474
                  tunnel: [w1518] -> w1473
                  tunnel: [w1514] -> w1472
                  tunnel: [w1513] -> w1471
                  tunnel: [w1517] -> w1470
                  tunnel: w1467 -> [w1520]
                  tunnel: w1465 -> [w1519]
                  tunnel: w1463 -> [w1518]
                  tunnel: w1461 -> [w1516]
                  tunnel: w1459 -> [w1513]
                  tunnel: w1457 -> [w1517]
                  tunnel: [w1511] -> w1456
                  tunnel: [w1535] -> w1488
                  tunnel: [w1534] -> w1487
                  tunnel: w1447 -> [w1532]
                  tunnel: [w1531] -> w1485
                  tunnel: [w1530] -> w1484
                  tunnel: [w1529] -> w1483
                  tunnel: w1482 -> [w1528]
                  tunnel: w1481 -> [w1527]
                  tunnel: w1480 -> [w1526]
                  tunnel: [w1525] -> w1479
                  tunnel: [w1524] -> w1478
                  tunnel: w1475 -> [w1539]
                  tunnel: w1474 -> [w1538]
                  tunnel: w1473 -> [w1537]
                  tunnel: w1472 -> [w1536]
                  tunnel: w1471 -> [w1533]
                  tunnel: w1470 -> [w1523]
                  tunnel: w1456 -> [w1521]
                  frame #0 {
                    # "Go to N subsite"
                    n429 = Number To Decimal String(number=w1494) -> (decimal integer string=w1495:string)  [unwired: 1 in]
                    n430 = Wait (ms)(milliseconds to wait=u32 1500) -> ()  [unwired: 1 out]
                    n431 = call "-mov-prob-abs-subs.vi"("Subsite #"=w1495) -> ()  [unwired: 5 in]
                  }
                  frame #1 {
                    n432 = call "Skip Current Subsite4"("Enable"=TRUE) -> ()  [unwired: 17 in, 2 out]
                    n433 = Wait (ms)(milliseconds to wait=u32 500) -> ()  [unwired: 1 out]
                  }
                  frame #2 {
                    n434 = local read "Bias Polarity"() -> (w1511:dbl)
                    n435 = call "Keith 237 Operate/Standby.vi"("source"=TRUE, "error in"=w1516, "GPIB address"=w1513) -> ("error out"=w1514:T2)
                    n436 = Wait (ms)(milliseconds to wait=u32 1000) -> ()  [unwired: 1 out]
                    n437 = local write "Status"("Starting CV Sensor Scan" ("Status")) -> ()
                  }
                  frame #3 {
                    w1522 = TRUE
                    n438 = while {
                      tunnel: w1533 -> [w1637]
                      tunnel: w1539 -> [w1564]
                      tunnel: w1538 -> [w1640]
                      tunnel: [w1622] -> w1534
                      tunnel: w1537 -> [w1623]
                      shift-right: [w1549] -> w1535
                      shift-left: w1536 -> [w1641]
                      tunnel: w1532 -> [w1635]
                      tunnel: [w1634] -> w1531
                      tunnel: [w1633] -> w1530
                      tunnel: [w1546] -> w1529
                      tunnel: w1528 -> [w1630]
                      tunnel: w1527 -> [w1628]
                      tunnel: w1526 -> [w1627]
                      tunnel: [w1626] -> w1525
                      tunnel: [w1611] -> w1524
                      tunnel: w1523 -> [w1569]
                      shift-right: [w1560] -> _
                      shift-left: w1522 -> [w1559]
                      shift-left: w1522 -> [w1543]
                      shift-left: w1522 -> [w1558]
                      shift-left: w1522 -> [w1542]
                      shift-left: w1522 -> [w1541]
                      tunnel: w1521 -> [w1540]
                      i -> [w1636]
                      stop <- w1553 continue-if-true
                      # "Only the K237 Bias and\nCapacitance are recorded in the \nXML file. The Excell file records \nK237 Bias, Capacitance, Secondary\nParameter, and Leakage Current\nas well as records the parameters\nset for the K237 and LCR meter"
                      # "Change Bias Polarity\n+1 Chuck Bias\n-1  Pad bias"
                      # "Plot Capacitance"
                      n439 = flat-sequence {
                        tunnel: w1623 -> [w1664]
                        tunnel: w1637 -> [w1665]
                        tunnel: w1641 -> [w1666]
                        tunnel: [w1666] -> w1598
                        tunnel: [w1665] -> w1597
                        tunnel: [w1664] -> w1596
                        tunnel: [w1663] -> w1576
                        tunnel: w1569 -> [w1662]
                        tunnel: w1634 -> [w1670]
                        tunnel: [w1671] -> w1595
                        tunnel: [w1669] -> w1593
                        tunnel: [w1668] -> w1591
                        tunnel: w1598 -> [w1672]
                        tunnel: w1597 -> [w1668]
                        tunnel: w1596 -> [w1669]
                        tunnel: [w1667] -> w1577
                        tunnel: w1576 -> [w1667]
                        tunnel: w1595 -> [w1677]
                        tunnel: [w1677] -> w1594
                        tunnel: w1593 -> [w1676]
                        tunnel: [w1676] -> w1592
                        tunnel: w1591 -> [w1675]
                        tunnel: [w1675] -> w1590
                        tunnel: w1577 -> [w1674]
                        tunnel: [w1673] -> w1574
                        tunnel: w1594 -> [w1682]
                        tunnel: [w1681] -> w1589
                        tunnel: [w1680] -> w1587
                        tunnel: w1592 -> [w1680]
                        tunnel: [w1679] -> w1585
                        tunnel: w1590 -> [w1679]
                        tunnel: [w1678] -> w1575
                        tunnel: w1574 -> [w1678]
                        tunnel: w1589 -> [w1687]
                        tunnel: [w1687] -> w1588
                        tunnel: w1587 -> [w1686]
                        tunnel: [w1686] -> w1586
                        tunnel: w1585 -> [w1685]
                        tunnel: [w1685] -> w1584
                        tunnel: w1575 -> [w1684]
                        tunnel: [w1683] -> w1570
                        tunnel: w1588 -> [w1690]
                        tunnel: w1586 -> [w1693]
                        tunnel: [w1689] -> w1610
                        tunnel: [w1693] -> w1609
                        tunnel: [w1692] -> w1608
                        tunnel: [w1691] -> w1607
                        tunnel: w1584 -> [w1691]
                        tunnel: [w1688] -> w1571
                        tunnel: w1570 -> [w1688]
                        tunnel: w1610 -> [w1705]
                        tunnel: [w1705] -> w1606
                        tunnel: w1609 -> [w1704]
                        tunnel: [w1704] -> w1605
                        tunnel: w1608 -> [w1703]
                        tunnel: [w1703] -> w1604
                        tunnel: w1607 -> [w1702]
                        tunnel: [w1702] -> w1603
                        tunnel: [w1700] -> w1572
                        tunnel: w1571 -> [w1700]
                        tunnel: w1606 -> [w1714]
                        tunnel: [w1714] -> w1583
                        tunnel: w1605 -> [w1713]
                        tunnel: [w1713] -> w1581
                        tunnel: w1604 -> [w1712]
                        tunnel: [w1712] -> w1579
                        tunnel: w1603 -> [w1707]
                        tunnel: [w1709] -> w1601
                        tunnel: [w1708] -> w1573
                        tunnel: w1572 -> [w1708]
                        tunnel: [w1707] -> w1565
                        tunnel: [w1706] -> w1561
                        tunnel: w1583 -> [w1719]
                        tunnel: [w1719] -> w1582
                        tunnel: w1581 -> [w1718]
                        tunnel: [w1718] -> w1580
                        tunnel: w1579 -> [w1717]
                        tunnel: [w1717] -> w1578
                        tunnel: w1573 -> [w1716]
                        tunnel: [w1715] -> w1566
                        tunnel: w1565 -> [w1715]
                        tunnel: w1582 -> [w1727]
                        tunnel: w1580 -> [w1726]
                        tunnel: w1578 -> [w1722]
                        tunnel: [w1727] -> w1621
                        tunnel: [w1726] -> w1620
                        tunnel: [w1722] -> w1619
                        tunnel: w1566 -> [w1720]
                        tunnel: [w1720] -> w1562
                        tunnel: w1621 -> [w1734]
                        tunnel: w1620 -> [w1733]
                        tunnel: w1619 -> [w1729]
                        tunnel: [w1734] -> w1618
                        tunnel: [w1733] -> w1617
                        tunnel: [w1729] -> w1616
                        tunnel: w1618 -> [w1741]
                        tunnel: w1617 -> [w1740]
                        tunnel: w1616 -> [w1739]
                        tunnel: [w1741] -> w1615
                        tunnel: [w1740] -> w1614
                        tunnel: [w1737] -> w1613
                        tunnel: [w1735] -> w1602
                        tunnel: [w1744] -> w1548
                        tunnel: [w1745] -> w1622
                        tunnel: [w1746] -> w1612
                        tunnel: w1615 -> [w1746]
                        tunnel: w1614 -> [w1745]
                        tunnel: w1613 -> [w1744]
                        tunnel: [w1742] -> w1552
                        tunnel: w1602 -> [w1742]
                        frame #0 {
                          n440 = call <vilib>:"Acquire Semaphore.vi"("semaphore"=w1662) -> ("semaphore out"=w1663:T1)  [unwired: 4 in, 2 out]
                        }
                        frame #1 {
                          # "Set Voltage"
                          n441 = call "Kei237_Set_Volt.vi"("Voltage"=w1670, "error in"=w1672, "GPIB"=w1668) -> ("error out"=w1671:errorcluster)
                        }
                        frame #2 {
                          n442 = call <vilib>:"Release Semaphore.vi"("semaphore"=w1674) -> ("semaphore out"=w1673:T1)  [unwired: 5 in, 1 out]
                        }
                        frame #3 {
                          n443 = call "Time Delay3"("error in (no error)"=w1682) -> ("error out"=w1681:errorcluster)  [unwired: 10 in]
                        }
                        frame #4 {
                          n444 = call <vilib>:"Acquire Semaphore.vi"("semaphore"=w1684) -> ("semaphore out"=w1683:T1)  [unwired: 4 in, 2 out]
                        }
                        frame #5 {
                          n445 = call "7000 Series Aquire Data.vi"("inst handle in"=w1693, "error in"=w1690) -> ("Primary"=w1694:string, "Primary Value"=w1695:string, "Primary Unit"=w1696:string, "Secondary"=w1699:string, "Secondary Value"=w1698:string, "Secondary Unit"=w1697:string, "error out"=w1689:T8)  [unwired: 5 in, 2 out]
                          n446 = Bundle("Primary"=w1694, "Primary Value"=w1695, "Primary Unit"=w1696, "Secondary"=w1699, "Secondary Value"=w1698, "Secondary Unit"=w1697) -> (w1692:T10)  [unwired: 1 in]
                        }
                        frame #6 {
                          n447 = Wait (ms)(milliseconds to wait=200) -> ()  [unwired: 1 out]
                        }
                        frame #7 {
                          n448 = call "K237-read-current-2.vi"("GPIB"=w1707) -> ("Current"=w1709:dbl)  [unwired: 1 in, 1 out]
                          "Compliance Level" <- w1709
                          n449 = local read "Compliance"() -> (w1710:dbl)
                          n450 = Absolute Value(x=w1709) -> (abs(x)=w1711:dbl)
                          n451 = Greater Or Equal?(x=w1711, y=w1710) -> (x >= y?=w1706:bool)
                          "Compliance" <- w1706
                        }
                        frame #8 {
                          n452 = call <vilib>:"Release Semaphore.vi"("semaphore"=w1716) -> ()  [unwired: 5 in, 2 out]
                        }
                        frame #9 {
                          n453 = Unbundle(w1722) -> ("Primary"=w1723:string, "Primary Unit"=w1724:string)  [unwired: 4 out]
                          n454 = call <vilib>:"Space Constant.vi"() -> ("String"=w1721:string)
                          n455 = Concatenate Strings(w1723, w1721, w1724) -> (w1725:string)
                          n456 = property on="Capacitance" class="XYGraph (strict)"("Caption.Text"=w1723, "YScale.NameLbl.Text"=w1725) -> ()  [unwired: 2 in, 2 out]
                        }
                        frame #10 {
                          n457 = call <vilib>:"Space Constant.vi"() -> ("String"=w1728:string)
                          n458 = Unbundle(w1729) -> ("Secondary"=w1731:string, "Secondary Unit"=w1730:string)  [unwired: 4 out]
                          n459 = Concatenate Strings(w1731, w1728, w1730) -> (w1732:string)
                          n460 = property on="Secondary Parameter Graph" class="XYGraph (strict)"("Caption.Text"=w1731, "YScale.NameLbl.Text"=w1732) -> ()  [unwired: 2 in, 2 out]
                        }
                        frame #11 {
                          n461 = Unbundle(w1739) -> ("Primary Value"=w1738:string, "Secondary Value"=w1736:string)  [unwired: 4 out]
                          n462 = Fract/Exp String To Number(string=w1738) -> (number=w1737:dbl)  [unwired: 3 in, 1 out]
                          n463 = Fract/Exp String To Number(string=w1736) -> (number=w1735:dbl)  [unwired: 3 in, 1 out]
                        }
                        frame #12 {
                          n464 = Wait (ms)(milliseconds to wait=200) -> ()  [unwired: 1 out]
                        }
                      }
                      n465 = Build Array(w1559, w1558, w1543, w1542, w1541) -> (w1557:bool[])
                      n466 = Multiply(x=w1640, y=w1636) -> (x*y=w1546:i32)
                      n467 = local write "K237_Bias"(w1546) -> ()
                      n468 = Multiply(x=w1540, y=w1546) -> (x*y=w1634:dbl)
                      n469 = Or Array Elements(Boolean array=w1557) -> (logical OR=w1554:bool)
                      n470 = Equal To 0?(x=w1636) -> (x = 0?=w1551:bool)
                      n471 = case shown="True" "Halt CV" {
                        selector: "Halt CV" -> [_ w1649]
                        tunnel: [FALSE ("source") w1650] -> w1632
                        tunnel: w1562 -> [_ w1645]
                        frame #0 {
                        }
                        frame #1 {
                          n472 = flat-sequence {
                            tunnel: w1649 -> [w1653]
                            tunnel: [w1653] -> w1648
                            tunnel: w1645 -> [w1651]
                            tunnel: [w1651] -> w1643
                            tunnel: w1648 -> [w1655]
                            tunnel: [w1656] -> w1647
                            tunnel: [w1654] -> w1644
                            tunnel: w1643 -> [w1654]
                            tunnel: w1647 -> [w1659]
                            tunnel: [w1659] -> w1646
                            tunnel: w1644 -> [w1657]
                            tunnel: [w1661] -> w1650
                            tunnel: w1646 -> [w1661]
                            frame #0 {
                              n473 = call "Keith 237 Operate/Standby.vi"("source"=FALSE, "GPIB address"=w1651) -> ()  [unwired: 1 in, 1 out]
                            }
                            frame #1 {
                              n474 = call "Prompt User for Input2"("Enable"=w1655) -> ("Yes"=w1656:bool)  [unwired: 17 in, 1 out]
                            }
                            frame #2 {
                              n475 = call "Keith 237 Operate/Standby.vi"("source"=TRUE, "GPIB address"=w1657) -> ()  [unwired: 1 in, 1 out]
                            }
                            frame #3 {
                              n476 = Wait (ms)(milliseconds to wait=750) -> ()  [unwired: 1 out]
                            }
                          }
                        }
                      }
                      n477 = Not(x=w1561) -> (.not. x?=w1560:bool)
                      n478 = Absolute Value(x=w1546) -> (abs(x)=w1625:i32)
                      n479 = Absolute Value(x=w1564) -> (abs(x)=w1624:i32)
                      n480 = Less?(x=w1625, y=w1624) -> (x < y?=w1555:bool)
                      n481 = Not(x=w1632) -> (.not. x?=w1556:bool)
                      n482 = Compound Arithmetic op=AND(w1554, w1555, w1556) -> (w1553:bool)
                      n483 = call "Primary"("error in (no error)"=w1612, "Reset"=w1551, "Y Input"=w1548, "X Input"=w1546) -> ("error out"=w1599:errorcluster, "XY Graph"=w1568:cluster{"Y":dbl[], "Y":dbl[]}[])  [unwired: 1 in, 5 out]
                      n484 = call "Secondary"("error in (no error)"=w1599, "Reset"=w1551, "Y Input"=w1552, "X Input"=w1546) -> ("error out"=w1550:errorcluster, "XY Graph"=w1567:cluster{"Y":dbl[], "Y":dbl[]}[])  [unwired: 1 in, 5 out]
                      n485 = Square(x=w1548) -> (x^2=w1547:dbl)
                      n486 = Reciprocal(x=w1547) -> (1/x=w1545:dbl)
                      n487 = call "1/C^2"("error in (no error)"=w1550, "Reset"=w1551, "Y Input"=w1545, "X Input"=w1546) -> ("error out"=w1549:errorcluster, "XY Graph"=w1544:cluster{"Y":dbl[], "Y":dbl[]}[])  [unwired: 1 in, 5 out]
                      n488 = local write "Secondary Parameter Graph"(w1567) -> ()
                      n489 = local write "1/C^2"(w1544) -> ()
                      n490 = Build Array(w1546, w1548) -> (w1631:dbl[])
                      n491 = Build Array(w1546, w1548, w1552, w1601, w1545) -> (w1600:dbl[])
                      n492 = call "XML_Data.vi"("Data Input Array"=w1631, "Data Tag Names Array"=w1627, "XML File Path"=w1628, "DOM document in"=w1630) -> ("DOM document out"=w1626:refnum<k20>)  [unwired: 6 in, 1 out]
                      n493 = call-poly <vilib>:"Write To Spreadsheet File.vi"("delimiter (\\t)"="," ("delimiter (\\t)"), "format (%.3f)"="%.3e" ("file format"), "append to file? (new file:F)"=TRUE, "1D data"=w1600, "file path (dialog if empty)"=w1635) -> ("new file path (Not A Path if cancelled)"=w1633:path)  [unwired: 2 in, 1 out]
                      n494 = local write "Capacitance"(w1568) -> ()
                      n495 = Bundle("XY Graph"=w1568, "XY Graph"=w1567, "XY Graph"=w1544) -> (w1611:T11)  [unwired: 1 in]
                    }
                  }
                }
                n496 = local write "Running Conditional"(TRUE) -> ()
                n497 = Open/Create/Replace File(file path (use dialog)=w1449, operation (0:open)=T5."replace or create", access (0:read/write)=enum16{"read/write", "read-only", "write-only"}."read/write") -> (refnum out=w1452:refnum<file>)  [unwired: 1 in, 4 out]
                n498 = Refnum to Path(1:w1452) -> (0:w1453:path)
                n499 = call-poly <vilib>:"Write To Spreadsheet File.vi"("delimiter (\\t)"="," ("delimiter (\\t)"), "append to file? (new file:F)"=FALSE, "2D data"=w1448, "file path (dialog if empty)"=w1453) -> ("new file path (Not A Path if cancelled)"=w1447:path)  [unwired: 4 in]
              }
              frame #1 {
                w1748 = cluster{"Y":dbl[], "Y":dbl[]}[] [] ("XY Graph")
                n500 = Bundle("XY Graph"=w1748, "XY Graph"=w1748, "XY Graph"=w1748) -> (w1754:T11)  [unwired: 1 in]
              }
            }
            n501 = Number To Fractional String(number=0) -> (F-format string=w1437:string)  [unwired: 3 in]
            n502 = Number To Fractional String(number=w1436) -> (F-format string=w1438:string)  [unwired: 3 in]
            n503 = Concatenate Strings(w1437, " : ", w1438) -> (→"Voltage Range":string)
            n504 = call-poly <vilib>:"Close.vi"("node"=w1428) -> ()  [unwired: 8 in, 1 out]
          }
          frame #2 {
            w1755 = FALSE
            # "The Parameters that are appended\nto the Excell file"
            n505 = property on="Primary Parameter" class="Ring (strict)"() -> ("RingText.Text"=w1771:string)  [unwired: 2 in, 2 out]
            n506 = property on="Secondary Parameter" class="Ring (strict)"() -> ("RingText.Text"=w1756:string)  [unwired: 2 in, 2 out]
            n507 = local read "Frequency"() -> (w1784:dbl)
            n508 = local read "Voltage Level"() -> (w1783:dbl)
            n509 = local read "CV-V-Steps"() -> (w1777:i32)
            n510 = local read "Voltage Range"() -> (w1772:string)
            n511 = local read "Number of Averages"() -> (w1776:dbl)
            n512 = local read "Time Delay mS"() -> (w1775:dbl)
            n513 = Number To Exponential String(number=w1784) -> (E-format string=w1781:string)  [unwired: 3 in]
            n514 = Number To Exponential String(number=w1783) -> (E-format string=w1780:string)  [unwired: 3 in]
            n515 = Number To Exponential String(number=w1777) -> (E-format string=w1779:string)  [unwired: 3 in]
            n516 = Number To Exponential String(number=w1776) -> (E-format string=w1778:string)  [unwired: 3 in]
            n517 = Number To Exponential String(number=w1775) -> (E-format string=w1773:string)  [unwired: 3 in]
            n518 = Build Array("LCR Parameters" ("element"), "Frequency", "Voltage Level", "Voltage Step", "Number of Averages", "Time Delay mS", "Voltage Range (K237)", "Primary", "Secondary") -> (w1763:string[])
            n519 = local write "Running Conditional"(w1755) -> ()
            n520 = local write "Running?"(w1755) -> ()
            n521 = Build Array("", w1781, w1780, w1779, w1778, w1773, w1772, w1771, w1756) -> (w1762:string[])
            n522 = Build Array(w1763, w1762) -> (w1761:string[][])
            n523 = call "Manual CV paramter_append.vi"("Array"=w1761, "Path"=w1760) -> ()  [unwired: 9 in, 1 out]
          }
          frame #3 {
            n524 = case shown="True" FALSE {
              tunnel: w1794 -> [w1797 w1802]
              tunnel: [w1797 w1801] -> w1793
              tunnel: w1792 -> [w1796 w1800]
              tunnel: [w1796 w1799] -> w1791
              tunnel: w1790 -> [_ w1798]
              frame #0 {
              }
              frame #1 {
                n525 = while {
                  tunnel: [w1818] -> w1799
                  tunnel: w1800 -> [w1812]
                  tunnel: w1802 -> [w1811]
                  tunnel: [w1811] -> w1801
                  tunnel: w1798 -> [w1805]
                  i -> [w1817]
                  stop <- w1814 continue-if-true
                  n526 = Multiply(x=25, y=w1817) -> (x*y=w1808:i32)
                  n527 = Sign(1:w1805) -> (0:w1810:i32)
                  n528 = Subtract(x=w1805, y=w1808) -> (x-y=w1807:i32)
                  n529 = Add(x=w1805, y=w1808) -> (x+y=w1806:i32)
                  n530 = Greater Than 0?(x=w1810) -> (x > 0?=w1809:bool)
                  n531 = Select(t=w1807, s=w1809, f=w1806) -> (s? t:f=w1803:i32)
                  n532 = Absolute Value(x=w1803) -> (abs(x)=w1804:i32)
                  n533 = local write "K237_Bias"(w1803) -> ()
                  n534 = call "Time Delay2"("error in (no error)"=w1812) -> ("error out"=w1813:errorcluster)  [unwired: 10 in]
                  n535 = Greater?(x=w1804, y=25) -> (0:w1814:bool)
                  n536 = call "Kei237_Set_Volt.vi"("Voltage"=w1803, "error in"=w1813, "GPIB"=w1811) -> ("error out"=w1818:errorcluster)
                }
              }
            }
          }
          frame #4 {
            n537 = Wait (ms)(milliseconds to wait=250) -> ()  [unwired: 1 out]
          }
          frame #5 {
            w1835 = 0
            n538 = In Range and Coerce(upper limit=3, x=w1829, lower limit=0) -> (In Range?=w1840:bool)  [unwired: 1 out]
            n539 = property on="Archive" class="TabCtl (strict)"("Value"=4) -> ()  [unwired: 2 in, 2 out]
            n540 = call "Kei237_Set_Volt.vi"("Voltage"=w1835, "error in"=w1845, "GPIB"=w1827) -> ("error out"=w1828:errorcluster)
            n541 = Wait Until Next ms Multiple(millisecond multiple=u32 250) -> ()  [unwired: 1 out]
            n542 = case shown="False" w1840 {
              tunnel: [w1867 0] -> w1839
              tunnel: w1829 -> [w1865 _]
              frame #0 {
                n543 = In Range and Coerce(upper limit=11, x=w1865, lower limit=4) -> (In Range?=w1866:bool)  [unwired: 1 out]
                n544 = case shown="False" w1866 {
                  tunnel: [2 1] -> w1867
                  frame #0 {
                  }
                  frame #1 {
                  }
                }
              }
              frame #1 {
              }
            }
            n545 = call "Keith 237 Operate/Standby.vi"("source"=FALSE, "error in"=w1828, "GPIB address"=w1827) -> ("error out"=w1825:T2)
            n546 = local write "K237_Bias"(w1835) -> ()
            n547 = Unbundle(w1833) -> (w1832:cluster{"Y":dbl[], "Y":dbl[]}[], w1831:cluster{"Y":dbl[], "Y":dbl[]}[], w1830:cluster{"Y":dbl[], "Y":dbl[]}[])
            n548 = local write "Status"("Finshing CV Sensor Scan" ("Status")) -> ()
            n549 = case shown="0, Default" w1839 {
              tunnel: [w1852 w1858 w1864] -> w1838
              tunnel: w1832 -> [w1851 w1858 w1864]
              tunnel: [w1850 w1857 w1863] -> w1837
              tunnel: w1831 -> [w1850 w1856 w1863]
              tunnel: [w1849 w1855 w1862] -> w1836
              tunnel: w1830 -> [w1849 w1855 w1861]
              tunnel: w1834 -> [w1848 w1854 w1860]
              frame #0 {
                # "Diodes"
                n550 = Unbundle(w1848) -> ("XY Graph"=w1847:cluster{"Y":dbl[], "Y":dbl[]}[])  [unwired: 2 out]
                n551 = Insert Into Array(array=w1851, new element=w1847) -> (w1852:cluster{"Y":dbl[], "Y":dbl[]}[])  [unwired: 1 in]
                "Diodes Capacitance" <- w1852
              }
              frame #1 {
                # "2x8s"
                n552 = Unbundle(w1854) -> ("XY Graph"=w1853:cluster{"Y":dbl[], "Y":dbl[]}[])  [unwired: 2 out]
                n553 = Insert Into Array(array=w1856, new element=w1853) -> (w1857:cluster{"Y":dbl[], "Y":dbl[]}[])  [unwired: 1 in]
                "2x8 Chip Capacitance" <- w1857
              }
              frame #2 {
                # "Single Chips"
                n554 = Unbundle(w1860) -> ("XY Graph"=w1859:cluster{"Y":dbl[], "Y":dbl[]}[])  [unwired: 2 out]
                n555 = Insert Into Array(array=w1861, new element=w1859) -> (w1862:cluster{"Y":dbl[], "Y":dbl[]}[])  [unwired: 1 in]
                "Single Chip Capacitance" <- w1862
              }
            }
          }
        }
        n556 = Concatenate Strings(w1325, "_CV.csv" ("string")) -> (w1366:string)
        n557 = Concatenate Strings(w1325, "_CV.xml" ("string")) -> (w1364:string)
        n558 = property on="Primary Parameter" class="Ring (strict)"() -> ("RingText.Text"=w1356:string)  [unwired: 2 in, 2 out]
        n559 = property on="Secondary Parameter" class="Ring (strict)"() -> ("RingText.Text"=w1353:string)  [unwired: 2 in, 2 out]
        n560 = Build Path(base path=w1363, name or relative path=w1366) -> (appended path=w1323:path)
        n561 = Build Array("Bias", w1356, w1353, "Leakage Current" ("element"), "1/C^2" ("element")) -> (w1381:string[])
        n562 = Build Path(base path=w1321, name or relative path=w1364) -> (appended path=w1362:path)
        n563 = Build Array(w1324, w1381) -> (w1322:string[][])
        n564 = Build Array("VOLTAGE_VOLT", "ACTV_CAP_FRD") -> (w1359:string[])
        n565 = call "XML_Initilize.vi"("User Input"=w1326) -> ("DOM document out"=w1368:refnum<k20>)  [unwired: 10 in]
      }
      n566 = call "7000 Series Configure.vi"("inst handle in"=w1315, "error in"=w1314, "Bias"=w1317) -> ("inst handle out"=w1316:refnum<visa-resource-name>, "error out"=w1312:T8)  [unwired: 22 in, 1 out]
      n567 = call "Keith 237 Reset.vi"("GPIB address"=w1313, "error in"=w1312) -> ("error out"=w1311:T2)
      n568 = call "7000 Series Close.vi"("error in (no error)"=w1311, "VISA session"=w1316) -> ("error out"=w1308:errorcluster)
    }
    frame #8 {
      n569 = local write "Stop Loop"(w1874) -> ()
      n570 = local write "Status"("Finished Full CV Scan" ("Status")) -> ()
      n571 = Wait (ms)(milliseconds to wait=u32 500) -> ()  [unwired: 1 out]
    }
    frame #9 {
      n572 = Build Array(16) -> (w1881:i32[])
      n573 = local write "Stop Loop"(TRUE ("Stop Loop")) -> ()
      n574 = EnableLocal(2:w1880, 3:w1881, 4:0) -> (0:→"error out":errorcluster)  [unwired: 1 out]
      n575 = local write "Status"("Full Automatic Scan Completed" ("Status")) -> ()
    }
  }
  n576 = call <vilib>:"Check if File or Folder Exists.vi"("path"=w24) -> ("file or folder exists?"=w23:bool, "dup path"=w22:path)  [unwired: 8 in, 1 out]
  n577 = case shown="False" w23 {
    tunnel: w22 -> [w1888 w1889]
    tunnel: [w1887 w1889] -> w4
    frame #0 {
      n578 = Create Folder(path (use dialog)=w1888) -> (created path=w1887:path)  [unwired: 2 in, 2 out]
    }
    frame #1 {
    }
  }
  n579 = while {
    tunnel: [w1891] -> _
    tunnel: w34 -> [w1891]
    stop <- "Stop Loop" continue-if-true
    n580 = call <vilib>:"Acquire Semaphore.vi"("semaphore"=w1891) -> ("semaphore out"=w1894:T1)  [unwired: 4 in, 2 out]
    n581 = Wait (ms)(milliseconds to wait=50) -> ()  [unwired: 1 out]
    n582 = case shown="True" "Emergency Stop" {
      selector: "Emergency Stop" -> [_ w1901]
      tunnel: w1894 -> [w1897 w1900]
      tunnel: [w1897 w1900] -> w1893
      tunnel: "IV or CV" -> [_ w1899]
      frame #0 {
      }
      frame #1 {
        n583 = case shown="0, Default" w1899 {
          tunnel: w1901 -> [w1903 w1963]
          tunnel: w1900 -> [w1902 w1962]
          frame #0 {
            n584 = flat-sequence {
              tunnel: [w1914] -> w1906
              tunnel: w1903 -> [w1914]
              tunnel: w1902 -> [w1911]
              tunnel: [w1911] -> w1905
              tunnel: w1906 -> [w1960]
              tunnel: [w1960] -> w1904
              tunnel: w1905 -> [w1959]
              tunnel: w1904 -> [w1961]
              frame #0 {
                n585 = flat-sequence {
                  tunnel: [w1915] -> w1912
                  tunnel: w1912 -> [w1921]
                  tunnel: [w1922] -> w1910
                  tunnel: [w1923] -> w1908
                  tunnel: w1910 -> [w1944]
                  tunnel: [w1944] -> w1909
                  tunnel: w1908 -> [w1943]
                  tunnel: [w1943] -> w1907
                  tunnel: [w1948] -> w1913
                  tunnel: w1909 -> [w1946]
                  tunnel: w1907 -> [w1945]
                  tunnel: w1913 -> [w1955]
                  frame #0 {
                    n586 = call "KE6485 Close.vi"("instrument handle"=refnum<k15> "GPIB0::10::INSTR") -> ("error out"=w1918:errorcluster)  [unwired: 10 in]
                    n587 = Wait (ms)(milliseconds to wait=2000) -> ()  [unwired: 1 out]
                    n588 = call "KE6485 Close.vi"("error in (no error)"=w1918, "instrument handle"=refnum<k15> "GPIB0::14::INSTR") -> ("error out"=w1915:errorcluster)  [unwired: 9 in]
                  }
                  frame #1 {
                    n589 = local read "K237_Bias"() -> (w1920:dbl)
                    n590 = while {
                      tunnel: [w1941] -> w1922
                      tunnel: "16" ("GPIB") -> [w1937]
                      tunnel: [w1937] -> w1923
                      shift-right: [w1926] -> _
                      shift-left: w1920 -> [w1932]
                      tunnel: w1921 -> [w1925]
                      i -> [w1928]
                      stop <- w1929 continue-if-true
                      n591 = Sign(1:w1932) -> (0:w1930:dbl)
                      n592 = Sign(1:w1928) -> (0:w1927:i32)
                      n593 = Greater Than 0?(x=w1930) -> (x > 0?=w1936:bool)
                      n594 = Multiply(x=25, y=w1927) -> (x*y=w1935:i32)
                      n595 = Subtract(x=w1932, y=w1935) -> (x-y=w1934:dbl)
                      n596 = Add(x=w1932, y=w1935) -> (x+y=w1933:dbl)
                      n597 = Select(t=w1934, s=w1936, f=w1933) -> (s? t:f=w1926:dbl)
                      n598 = Absolute Value(x=w1926) -> (abs(x)=w1931:dbl)
                      n599 = call "Time Delay5"("error in (no error)"=w1925) -> ("error out"=w1938:errorcluster)  [unwired: 10 in]
                      n600 = Greater?(x=w1931, y=25) -> (0:w1929:bool)
                      n601 = call "Kei237_Set_Volt.vi"("Voltage"=w1926, "error in"=w1938, "GPIB"=w1937) -> ("error out"=w1941:errorcluster)
                    }
                  }
                  frame #2 {
                    n602 = Wait (ms)(milliseconds to wait=750) -> ()  [unwired: 1 out]
                  }
                  frame #3 {
                    n603 = call "Kei237_Set_Volt.vi"("Voltage"=0, "error in"=w1946, "GPIB"=w1945) -> ("error out"=w1950:errorcluster)
                    n604 = call "Keith 237 Reset.vi"("GPIB address"=w1945, "error in"=w1950) -> ("error out"=w1948:T2)
                    n605 = Wait (ms)(milliseconds to wait=750) -> ()  [unwired: 1 out]
                  }
                  frame #4 {
                    n606 = Build Array(16, 10, 14) -> (w1951:i32[])
                    n607 = EnableLocal(2:w1955, 3:w1951, 4:0) -> (0:→"error out 6":errorcluster)  [unwired: 1 out]
                  }
                }
              }
              frame #1 {
                w1958 = FALSE ("Emergency Stop")
                n608 = local write "Emergency Stop"(w1958) -> ()
                n609 = local write "Bias Loop"(w1958) -> ()
                n610 = call <vilib>:"Release Semaphore Reference.vi"("semaphore"=w1959) -> ()  [unwired: 9 in, 2 out]
              }
              frame #2 {
                n611 = Stop(stop? (T)=w1961) -> ()
              }
            }
          }
          frame #1 {
            n612 = flat-sequence {
              tunnel: [w1974] -> w1966
              tunnel: w1963 -> [w1974]
              tunnel: w1962 -> [w1972]
              tunnel: [w1972] -> w1965
              tunnel: w1966 -> [w2019]
              tunnel: [w2019] -> w1964
              tunnel: w1965 -> [w2018]
              tunnel: w1964 -> [w2020]
              frame #0 {
                n613 = flat-sequence {
                  tunnel: [w1978] -> w1971
                  tunnel: [w1983] -> w1970
                  tunnel: [w1984] -> w1968
                  tunnel: w1971 -> [w1981]
                  tunnel: w1970 -> [w2005]
                  tunnel: [w2005] -> w1969
                  tunnel: w1968 -> [w2004]
                  tunnel: [w2004] -> w1967
                  tunnel: [w2009] -> w1973
                  tunnel: w1969 -> [w2006]
                  tunnel: w1967 -> [w2007]
                  tunnel: w1973 -> [w2014]
                  frame #0 {
                    w1976 = u16 0 items=["Off", "Internal", "External"] ("Bias")
                    n614 = call "7000 Series Configure.vi"("inst handle in"=refnum<visa-resource-name> "GPIB0::4::INSTR", "Bias"=w1976) -> ("inst handle out"=w1980:refnum<visa-resource-name>, "error out"=w1979:T8)  [unwired: 23 in, 1 out]
                    n615 = Wait (ms)(milliseconds to wait=2000) -> ()  [unwired: 1 out]
                    n616 = call "7000 Series Close.vi"("error in (no error)"=w1979, "VISA session"=w1980) -> ("error out"=w1978:errorcluster)
                  }
                  frame #1 {
                    n617 = local read "K237_Bias"() -> (w1982:dbl)
                    n618 = while {
                      tunnel: [w2002] -> w1983
                      tunnel: "16" ("GPIB") -> [w1998]
                      tunnel: [w1998] -> w1984
                      shift-right: [w1987] -> _
                      shift-left: w1982 -> [w1993]
                      tunnel: w1981 -> [w1986]
                      i -> [w1989]
                      stop <- w1990 continue-if-true
                      n619 = Sign(1:w1993) -> (0:w1991:dbl)
                      n620 = Sign(1:w1989) -> (0:w1988:i32)
                      n621 = Greater Than 0?(x=w1991) -> (x > 0?=w1997:bool)
                      n622 = Multiply(x=25, y=w1988) -> (x*y=w1996:i32)
                      n623 = Subtract(x=w1993, y=w1996) -> (x-y=w1995:dbl)
                      n624 = Add(x=w1993, y=w1996) -> (x+y=w1994:dbl)
                      n625 = Select(t=w1995, s=w1997, f=w1994) -> (s? t:f=w1987:dbl)
                      n626 = Absolute Value(x=w1987) -> (abs(x)=w1992:dbl)
                      n627 = call "Time Delay6"("error in (no error)"=w1986) -> ("error out"=w1999:errorcluster)  [unwired: 10 in]
                      n628 = Greater?(x=w1992, y=25) -> (0:w1990:bool)
                      n629 = call "Kei237_Set_Volt.vi"("Voltage"=w1987, "error in"=w1999, "GPIB"=w1998) -> ("error out"=w2002:errorcluster)
                    }
                  }
                  frame #2 {
                    n630 = Wait (ms)(milliseconds to wait=750) -> ()  [unwired: 1 out]
                  }
                  frame #3 {
                    n631 = call "Kei237_Set_Volt.vi"("Voltage"=0, "error in"=w2006, "GPIB"=w2007) -> ("error out"=w2011:errorcluster)
                    n632 = Wait (ms)(milliseconds to wait=750) -> ()  [unwired: 1 out]
                    n633 = call "Keith 237 Reset.vi"("GPIB address"=w2007, "error in"=w2011) -> ("error out"=w2009:T2)
                  }
                  frame #4 {
                    n634 = Build Array(16) -> (w2012:i32[])
                    n635 = EnableLocal(2:w2014, 3:w2012, 4:0) -> (0:→"error out 7":errorcluster)  [unwired: 1 out]
                  }
                }
              }
              frame #1 {
                w2017 = FALSE ("Emergency Stop")
                n636 = local write "Emergency Stop"(w2017) -> ()
                n637 = local write "Bias Loop"(w2017) -> ()
                n638 = call <vilib>:"Release Semaphore Reference.vi"("semaphore"=w2018) -> ()  [unwired: 9 in, 2 out]
              }
              frame #2 {
                n639 = Stop(stop? (T)=w2020) -> ()
              }
            }
          }
        }
        n640 = local write "Status"("Emergency Stop" ("Status")) -> ()
      }
    }
    n641 = call <vilib>:"Release Semaphore.vi"("semaphore"=w1893) -> ()  [unwired: 5 in, 2 out]
  }
  n642 = Build Path(base path=w4, name or relative path=w3) -> (appended path=w2:path)
  n643 = call <vilib>:"Check if File or Folder Exists.vi"("path"=w2) -> ("file or folder exists?"=w6:bool, "dup path"=w5:path)  [unwired: 8 in, 1 out]
  n644 = case shown="False" w6 {
    tunnel: w5 -> [w2022 w2023]
    tunnel: [w2021 w2023] -> w1
    frame #0 {
      n645 = Create Folder(path (use dialog)=w2022) -> (created path=w2021:path)  [unwired: 2 in, 2 out]
    }
    frame #1 {
    }
  }
  n646 = Build Path(base path=w1, name or relative path="XML") -> (appended path=w8:path)
  n647 = call <vilib>:"Check if File or Folder Exists.vi"("path"=w8) -> ("file or folder exists?"=w11:bool, "dup path"=w10:path)  [unwired: 8 in, 1 out]
  n648 = case shown="False" w11 {
    tunnel: w10 -> [w2025 w2026]
    tunnel: [w2024 w2026] -> w7
    frame #0 {
      n649 = Create Folder(path (use dialog)=w2025) -> (created path=w2024:path)  [unwired: 2 in, 2 out]
    }
    frame #1 {
    }
  }
  n650 = while {
    tunnel: ["Bias Loop"] -> w60
    stop <- "Bias Loop" stop-if-true
    n651 = Wait (ms)(milliseconds to wait=250) -> ()  [unwired: 1 out]
    n652 = case shown="True" "Running Conditional" {
      frame #0 {
        n653 = local write "Running?"(FALSE ("Running?")) -> ()
      }
      frame #1 {
        "Running?" <- TRUE
      }
    }
  }
  n654 = local write "Compliance"(w48) -> ()
  n655 = local write "Bias Loop"(w47) -> ()
  n656 = Not(x=w60) -> (.not. x?=w59:bool)
  n657 = local write "Bias Loop"(w59) -> ()
